vi "EC_Applied_Motion_SXSYSZ_20170419A_3chNoBKorg.vi"() -> ()   [LabVIEW 2015]
uses:
  <vilib>/Instr/_visa.llb/VISA Configure Serial Port (Instr).vi
  <userlib>/caLab/Private/Put_DBL-1D_PV-1D.vi
  <vilib>/Utility/file.llb/Write To Spreadsheet File (I64).vi
  <vilib>/Utility/file.llb/Read From Spreadsheet File (I64).vi
panel:
  in  "GFS":bool=TRUE
  out "NC":bool
  in  "Override 2":bool
  out "Dev5 Voltage 2":dbl
  out "Dev5 Voltage":dbl
  in  "Override":bool
  in  "APX:FZabs":dbl
  in  "Move Z":bool
  in  "Jog Z-":bool
  in  "Jog X-":bool
  in  "Jog Y-":bool
  out "Z Velocity MV mm/sec":dbl format="%.3f"
  out "Z Position MV mm":dbl
  out "Y Velocity MV mm/sec":dbl format="%.3f"
  out "Y Position MV mm":dbl
  out "X Velocity MV mm/sec":dbl format="%.3f"
  out "X Position MV mm":dbl
  in  "stop":bool
  in  "Tab Control 3":enum32{"Status", "Reset"}(tab)
  out "Y in Range":bool
  out "Y in Motion":bool
  out "X  in Range":bool
  out "X  in Motion":bool
  out "Z in Range":bool
  out "Z in Motion":bool
  out "X Ready":bool
  out "Y Ready":bool
  out "Z Ready":bool
  in  "Reset Y Position mm":dbl
  out "Reset Y Motor Steps":i32
  in  "Reset X Position mm":dbl
  out "Reset X Motor Steps":i32
  in  "Reset Z Position mm":dbl
  out "Reset Z Motor Steps":i32
  in  "Reset":bool
  in  "Tab Control":enum32{"mm", "preset", "step"}(tab)
  in  "APX:FXstep":dbl
  in  "FX Velocity SP mm/sec":dbl=0.01
  in  "APX:FYstep":dbl
  in  "FY Velocity SP mm/sec":dbl=0.01
  in  "APX:Fzstep":dbl
  in  "FZ Velocity SP mm/sec":dbl=0.01
  in  "Z Jog Set":bool
  in  "Y Jog Set":bool
  in  "X Jog Set":bool
  in  "X Velocity SP step/sec":i32 min=1 max=1000
  in  "Y Velocity SP step/sec":i32 min=1 max=1000
  in  "Z Velocity SP step/sec":i32 min=1 max=500
  in  "Y Step SP":i32=-20000 min=-800000 max=800000 step=500
  in  "X Step SP":i32=-20000 min=-750000 max=750000 step=500
  in  "Z Step SP":i32=-20000 min=-3000 max=102400000 step=500
  out "X Step PV":i32 max=2000
  out "Y Step PV":i32 max=2000
  out "Z Step PV":i32 max=2000
  out "R Step PV":i32 max=2000
  in  "Z Abso SP":i32=-20000 min=-3000 max=102400000 step=500
  out "Z COM PORT":refnum<visa-resource-name>="COM5"
  out "Z Holding Current %":i32
  out "Z Run Current %":i32
  out "Z offset mm":dbl
  out "Z mm/rev":dbl
  out "Z steps/rev":u32
  out "Z  velocity PV step/sec":i32
  out "Z MINPOS":i32=-94296
  out "Z MAXPOS":i32=-34296
  in  "Jog Z+":bool
  out "Z Position mm PV":dbl
  out "X Position mm PV":dbl
  out "X velocity PV step/sec":i32
  in  "Jog X+":bool
  out "X Holding Current %":i32
  out "X Run Current %":i32
  out "X offset mm":dbl
  out "X mm/rev":dbl
  out "X steps/rev":u32
  out "X MAXPOS":i32=-34296
  out "X MINPOS":i32=-94296
  out "X COM PORT":refnum<visa-resource-name>="COM5"
  out "Y Holding Current %":i32
  out "Y Run Current %":i32
  out "Y Position mm PV":dbl
  out "Y offset mm":dbl
  out "Y mm/rev":dbl
  out "Y steps/rev":u32
  out "Y velocity PV step/sec":i32
  in  "Stop":bool
  in  "Jog Y+":bool
  out "Y MINPOS":i32=-94296
  out "Y MAXPOS":i32=-34296
  out "Y COM PORT":refnum<visa-resource-name>="COM5"
  # "APX:FY"
  # "x-ray"
  # "APX:FZ"
  # "APX:FX"
  # "SPEAR"
  # "APX:FinePos"
  # "Stage"
  # "Current position"
  # "Jog step/velovity"
  # "sample to SSRL"
  # "FX"
  # "FY"
  # "FZ"
  # "R,L = green"
  # "L"
  # "M"
  # "B"
  # "S"
  # "R"
  # "Preset position"
types:
  T1 = enum16{"Power-up Signature", "Accel Rate", "Accel Max", "Bit Rate", "Buffer Status", "Change Current", "Commence Jogging", "Change Jog Speed", "Continue", "Define Address", "Distance for FC,FM,FO,FY", "Decel Rate", "Distance or Position", "Define Limits", "Encoder Deadband", "Encoder Function", "Encoder Position", "Encoder Ratio", "Feed to Length with Speed Change", "Feed to Length", "Feed to Sensor with Mask Dist", "Feed to Length & Set Output", "Feed to Position", "Feed to Sensor", "Feed to Sensor w/safety", "Follow Handwheel", "Immediate Distance?", "Immediate Encoder?", "Immediate Low Output", "Immediate High Output", "Immediate Position?", "Input Status?", "Jog Accel/Decel", "Jog Disable", "Jog Enable", "Jog Speed", "Motor Disable", "Motor Enable", "Microstep Resolution", "Power up Current", "Power up Mode", "Pause", "Request Status", "Revision Level?", "Seek Home", "Stop Jogging", "Stop & Kill Buffer", "Set Output", "Set ABS Position", "Send String", "Stop", "Velocity for Speed Change", "Velocity Setting", "Wait for Input", "Wait Time"}
  T2 = enum8{"Enabled", "Disabled", "Disabled and Grayed Out"}
  T3 = cluster{"first row[0]":i64, "first row[1]":i64, "first row[2]":i64, "first row[3]":i64, "first row[4]":i64, "first row[5]":i64, "first row[6]":i64, "first row[7]":i64, "first row[8]":i64}
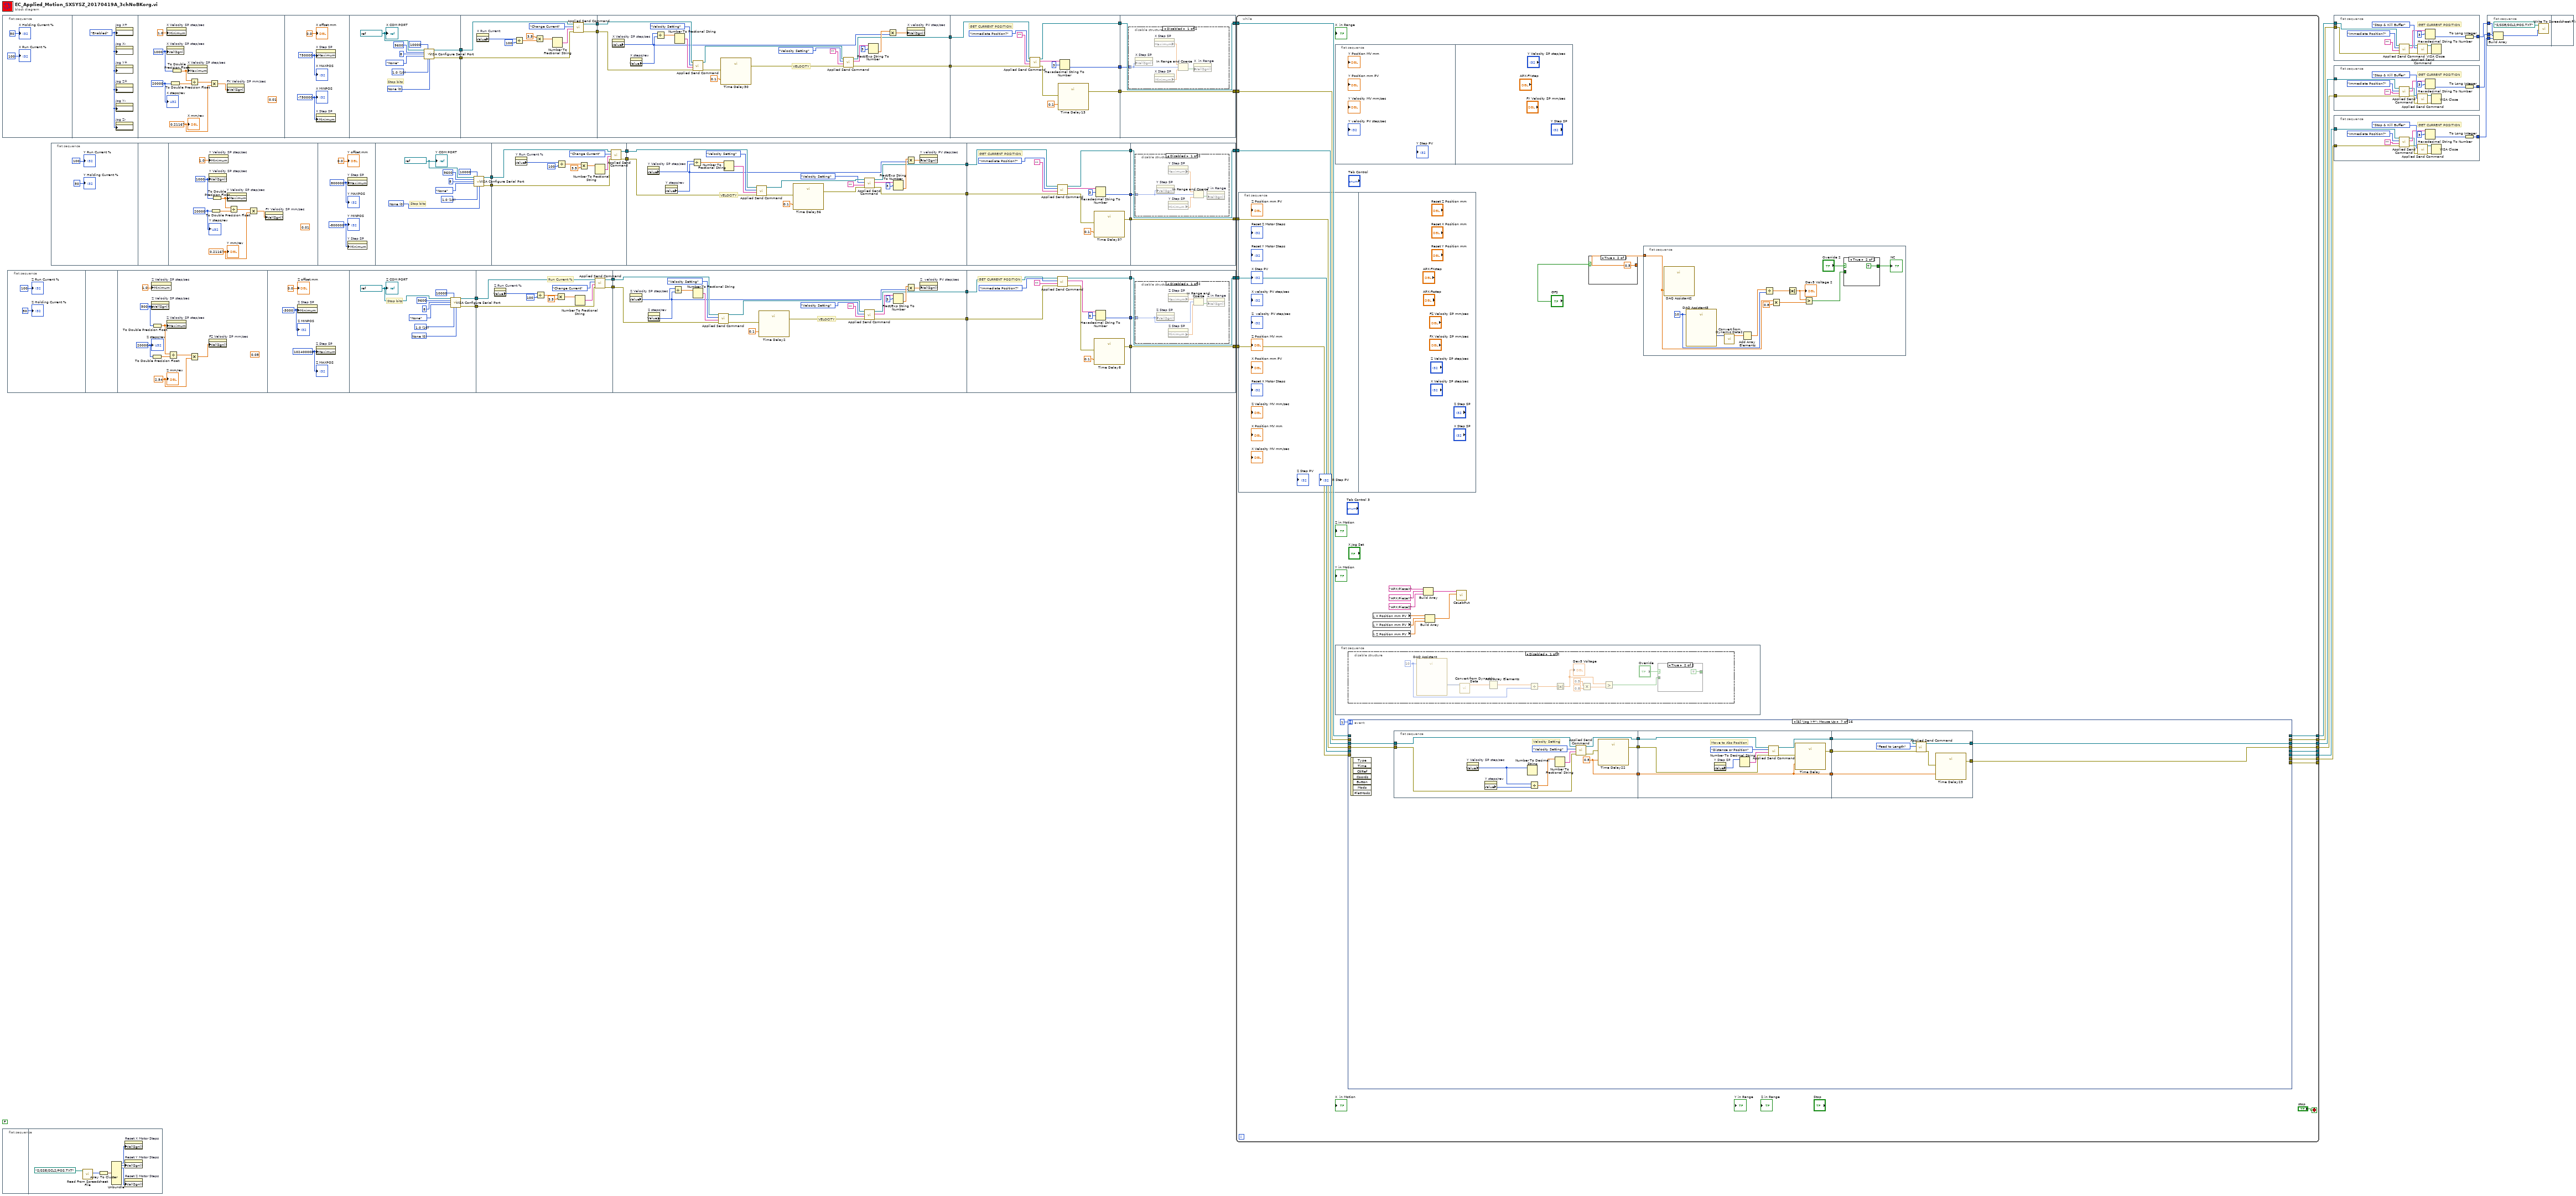
[diagram p0: block diagram]
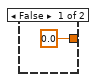
[diagram p5: hidden frame]
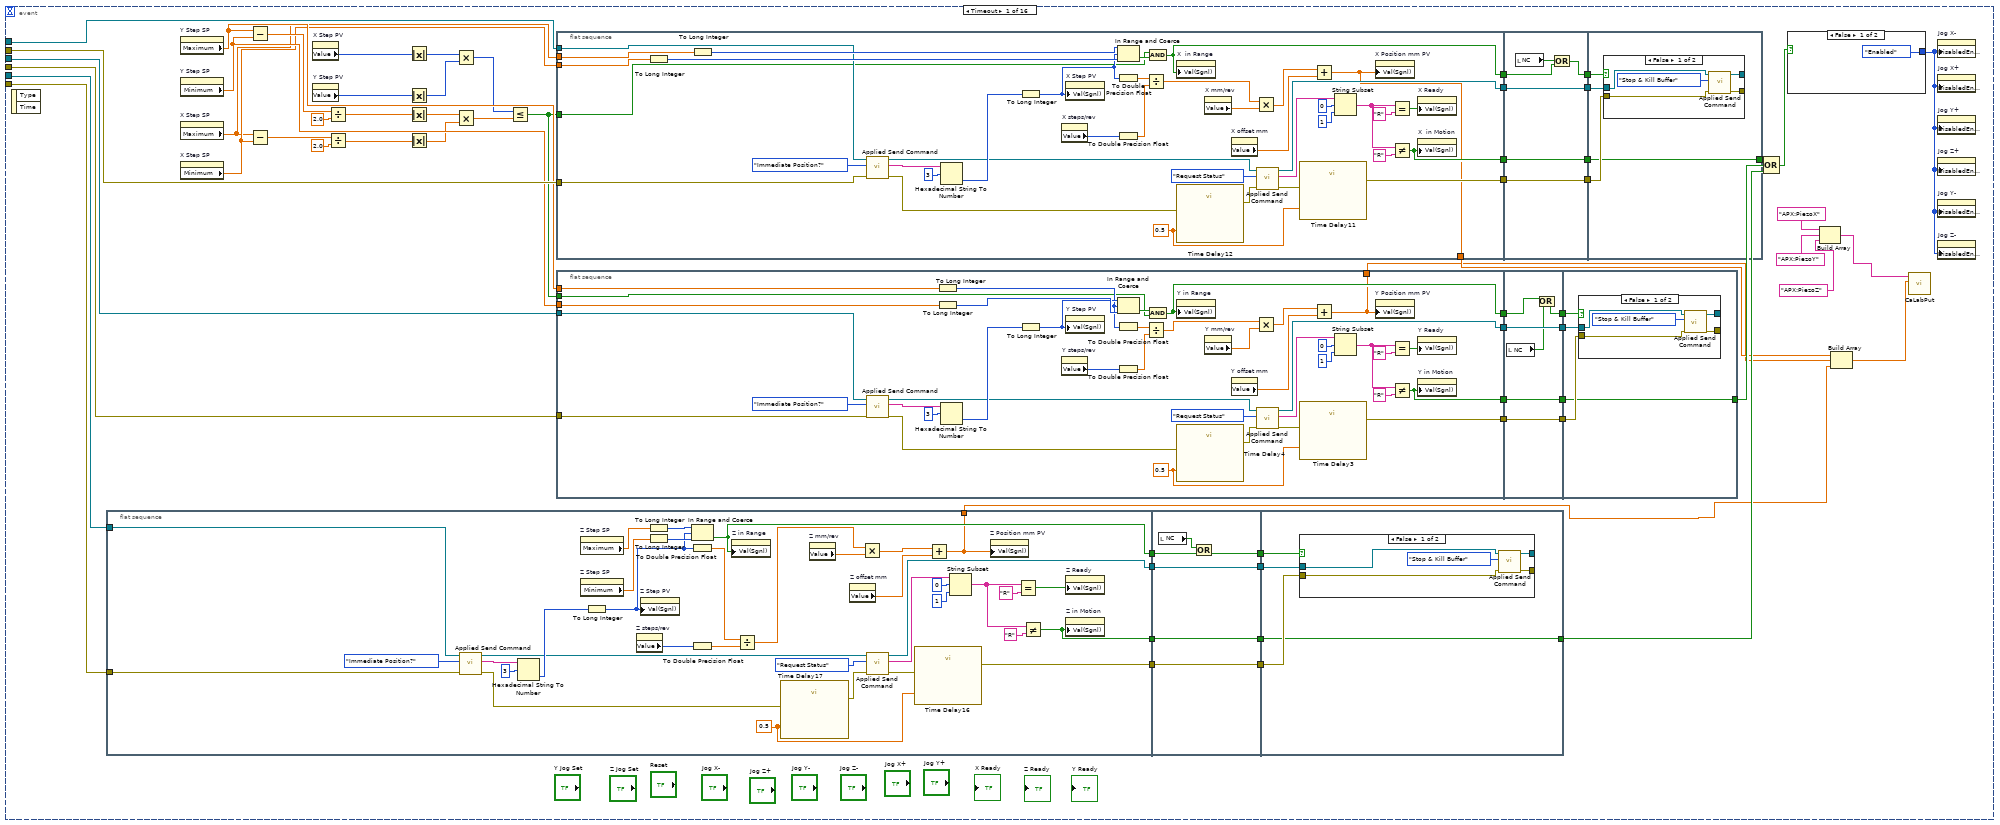
[diagram p9: hidden frame]
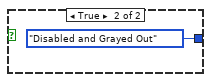
[diagram p10: hidden frame]
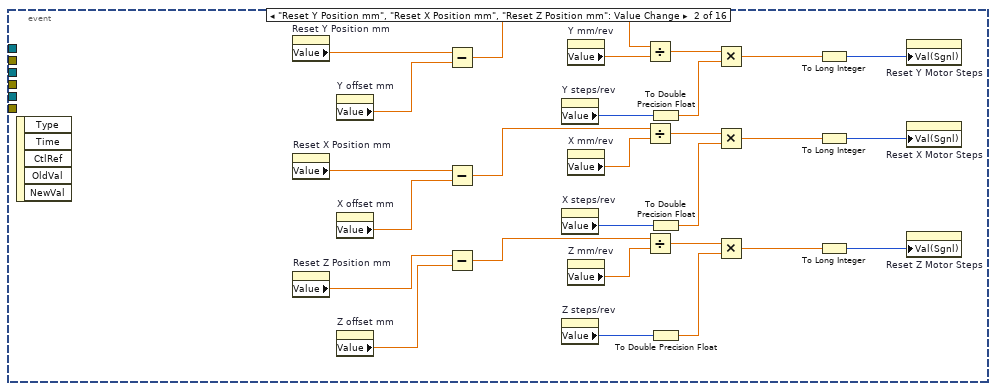
[diagram p14: hidden frame]
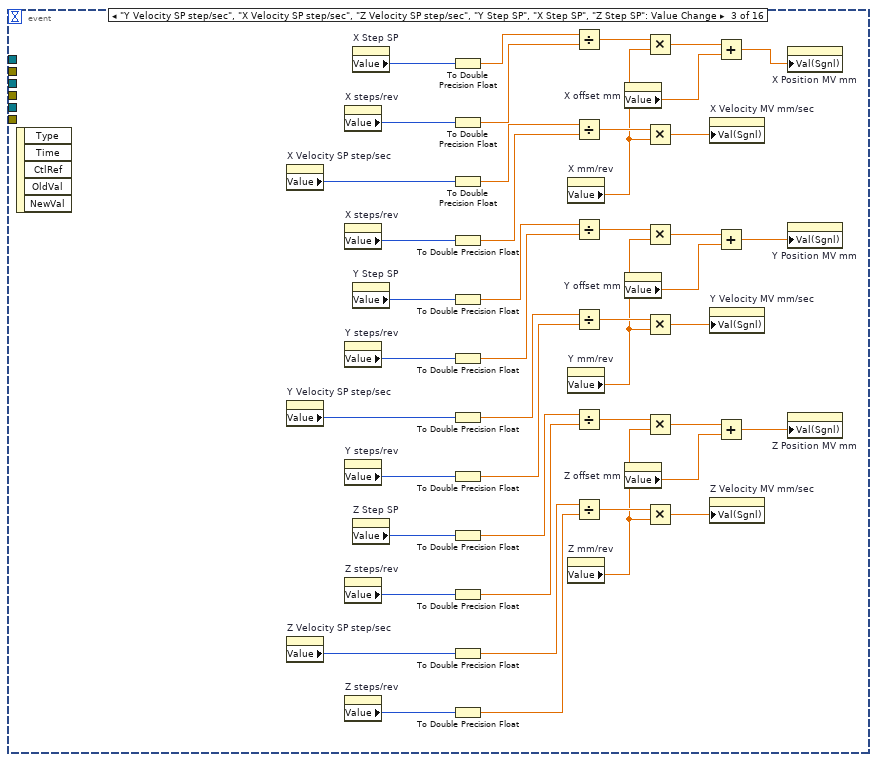
[diagram p15: hidden frame]
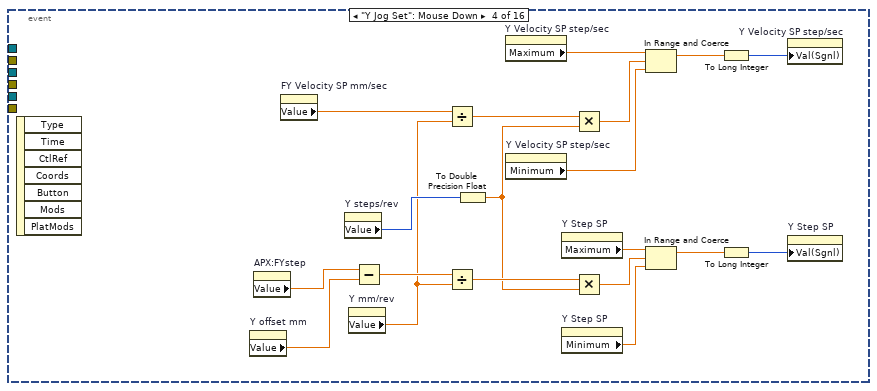
[diagram p16: hidden frame]
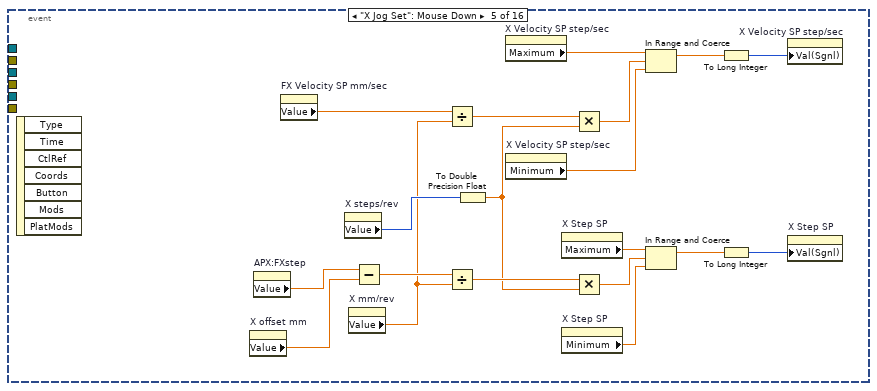
[diagram p17: hidden frame]
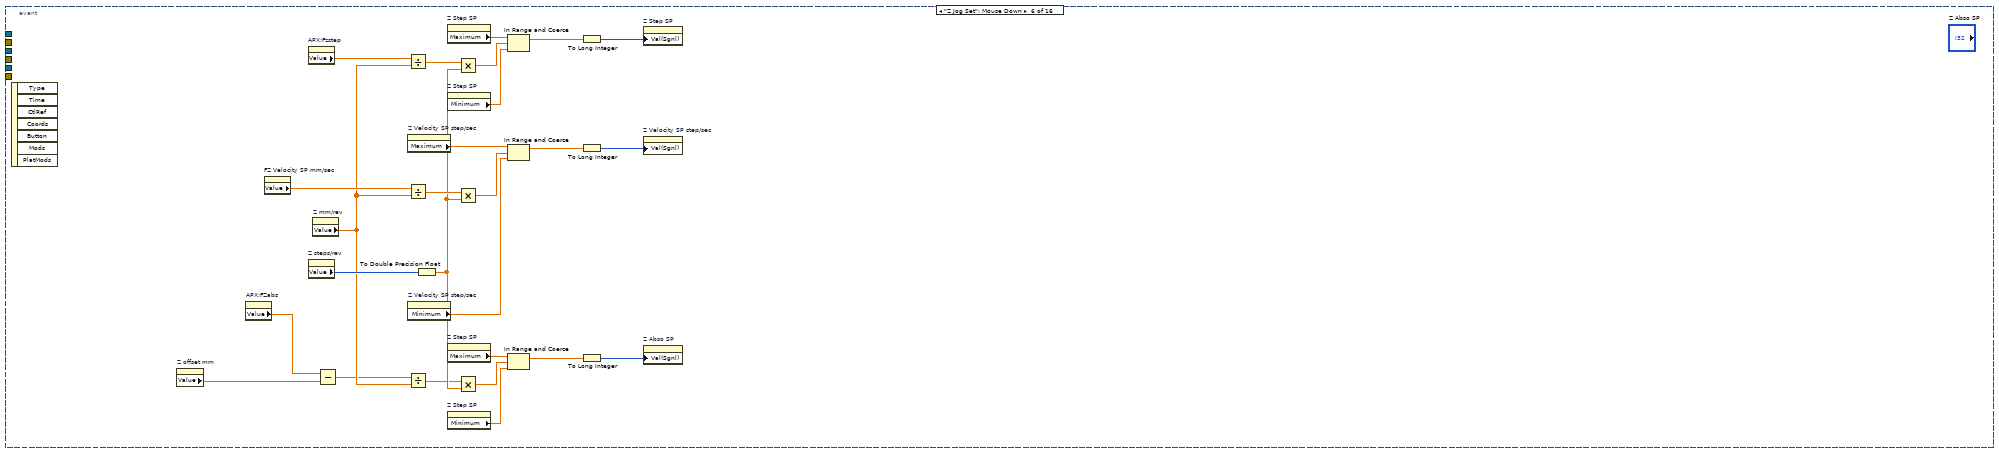
[diagram p18: hidden frame]
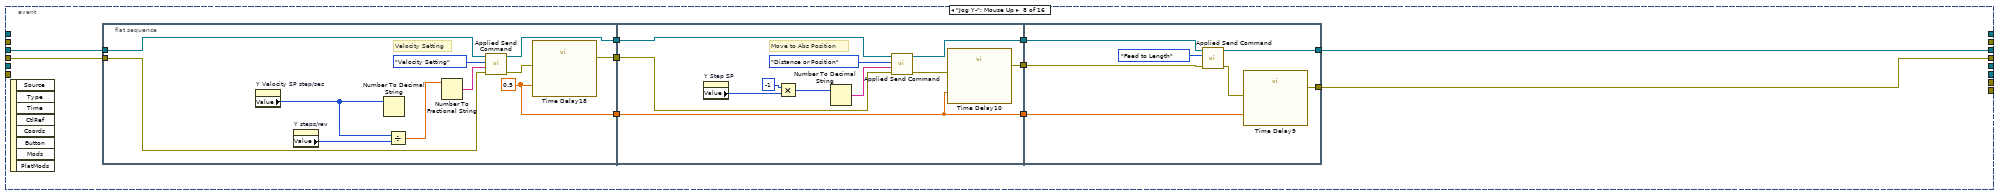
[diagram p19: hidden frame]
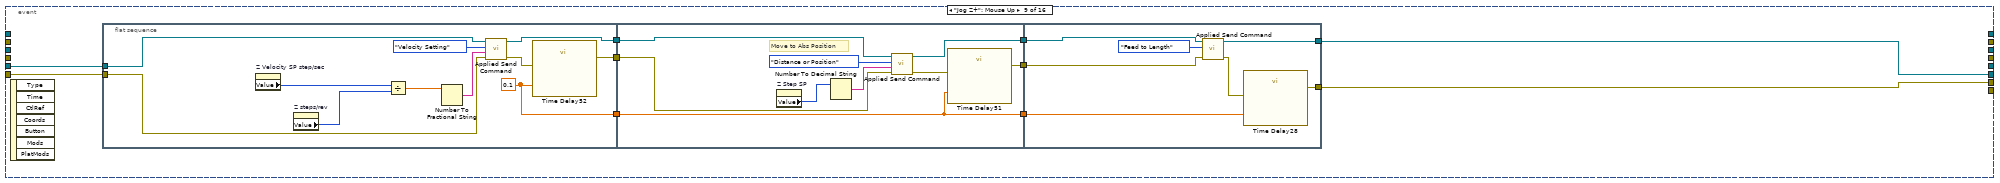
[diagram p20: hidden frame]
diagram:
  (unwired) FALSE
  n1 = flat-sequence {
    tunnel: [w58] -> w18
    tunnel: [w57] -> w17
    tunnel: w18 -> [w75]
    tunnel: w17 -> [w74]
    tunnel: [w73] -> w16
    tunnel: [w72] -> w15
    tunnel: [w78] -> w40
    tunnel: w16 -> [w86]
    tunnel: w15 -> [w85]
    tunnel: [w79] -> w14
    tunnel: w40 -> [w100]
    tunnel: [w99] -> w34
    tunnel: [w97] -> w33
    tunnel: [w102] -> w32
    tunnel: w14 -> [w101]
    tunnel: [w108] -> w38
    tunnel: [w109] -> w39
    tunnel: w34 -> [w109]
    tunnel: w33 -> [w108]
    tunnel: w32 -> [w107]
    frame #0 {
      "X Run Current %" <- 100 ("Run Current %")
      "X Holding Current %" <- 50 ("Holding Current %")
    }
    frame #1 {
      w45 = T2."Enabled" ("Disabled")
      n2 = property on="Jog X+" class="Bool"("DisabledEnum"=w45) -> ()  [unwired: 2 in, 2 out]
      n3 = property on="Jog X-" class="Bool"("DisabledEnum"=w45) -> ()  [unwired: 2 in, 2 out]
      n4 = property on="Jog Y+" class="Bool"("DisabledEnum"=w45) -> ()  [unwired: 2 in, 2 out]
      n5 = property on="Jog Z+" class="Bool"("DisabledEnum"=w45) -> ()  [unwired: 2 in, 2 out]
      n6 = property on="Jog Y-" class="Bool"("DisabledEnum"=w45) -> ()  [unwired: 2 in, 2 out]
      n7 = property on="Jog Z-" class="Bool"("DisabledEnum"=w45) -> ()  [unwired: 2 in, 2 out]
    }
    frame #2 {
      w48 = 0.21167 ("MM/rev")
      w51 = u32 20000 ("step/rev")
      w46 = 1000 ("Value (Signaling)")
      (unwired) 0.01 ("Value (Signaling)")
      n8 = property on="X Velocity SP step/sec" class="DigNum (strict)"("Minimum"=1.0 ("Data Entry Limits:Minimum")) -> ()  [unwired: 2 in, 2 out]
      n9 = property on="X Velocity SP step/sec" class="DigNum (strict)"("Val(Sgnl)"=w46) -> ()  [unwired: 2 in, 2 out]
      n10 = To Double Precision Float(number=w51) -> (double precision float=w50:dbl)
      n11 = To Double Precision Float(number=w46) -> (double precision float=w52:dbl)
      n12 = property on="X Velocity SP step/sec" class="DigNum (strict)"("Maximum"=w52) -> ()  [unwired: 2 in, 2 out]
      n13 = Divide(x=w52, y=w50) -> (x/y=w47:dbl)
      n14 = Multiply(x=w47, y=w48) -> (x*y=w49:dbl)
      n15 = property on="FX Velocity SP mm/sec" class="DigNum (strict)"("Val(Sgnl)"=w49) -> ()  [unwired: 2 in, 2 out]
      "X steps/rev" <- w51
      "X mm/rev" <- w48
    }
    frame #3 {
      w56 = -750000 ("lower limit")
      w55 = 750000 ("upper limit")
      n16 = property on="X Step SP" class="DigNum (strict)"("Maximum"=w55) -> ()  [unwired: 2 in, 2 out]
      n17 = property on="X Step SP" class="DigNum (strict)"("Minimum"=w56) -> ()  [unwired: 2 in, 2 out]
      "X offset mm" <- 0.0 ("offset")
      "X MAXPOS" <- w55
      "X MINPOS" <- w56
    }
    frame #4 {
      w65 = refnum<visa-resource-name> "COM21" ("COM PORT")
      w63 = u16 0 items=["None", "XON/XOFF", "RTS/CTS", "XON/XOFF & RTS/CTS", "DTR/DSR", "XON/XOFF & DTR/DSR"] ("flow control (0:none)")
      w62 = u16 10 items=["1.0"=10, "1.5"=15, "2.0"=20] ("stop bits (10: 1 bit)")
      # "Stop bits"
      n18 = call-poly "VISA Configure Serial Port"("VISA resource name"=w65, "timeout (10sec)"=u32 10000, "baud rate (9600)"=u32 9600, "data bits (8)"=u16 8, "parity (0:none)"=enum16{"None", "Odd", "Even", "Mark", "Space"}."None", "stop bits (10: 1 bit)"=w62, "flow control (0:none)"=w63) -> ("VISA resource name out"=w58:refnum<visa-resource-name>, "error out"=w57:errorcluster)  [unwired: 7 in]
      "X COM PORT" <- w65
    }
    frame #5 {
      n19 = property on="X Run Current" class="DigNum (strict)"() -> ("Value"=w70:i32)  [unwired: 2 in, 2 out]
      n20 = Divide(x=w70, y=100) -> (x/y=w67:dbl)
      n21 = Multiply(x=3.5 ("y"), y=w67) -> (x*y=w69:dbl)
      n22 = Number To Fractional String(number=w69) -> (F-format string=w71:string)  [unwired: 3 in]
      n23 = call "Applied Send Command.vi"("error in (no error)"=w74, "Extra"=w71, "Command"=T1."Change Current", "VISA resource name"=w75) -> ("error out"=w73:errorcluster, "VISA resource name out"=w72:refnum<visa-resource-name>)  [unwired: 3 in, 1 out]
    }
    frame #6 {
      # "VELOCITY"
      n24 = property on="X Velocity SP step/sec" class="DigNum (strict)"() -> ("Value"=w82:i32)  [unwired: 2 in, 2 out]
      n25 = property on="X steps/rev" class="DigNum (strict)"() -> ("Value"=w81:u32)  [unwired: 2 in, 2 out]
      n26 = Divide(x=w82, y=w81) -> (x/y=w80:dbl)
      n27 = Number To Fractional String(number=w80) -> (F-format string=w87:string)  [unwired: 3 in]
      n28 = call "Applied Send Command.vi"("error in (no error)"=w86, "Extra"=w87, "Command"=T1."Velocity Setting", "VISA resource name"=w85) -> ("error out"=w88:errorcluster, "VISA resource name out"=w95:refnum<visa-resource-name>)  [unwired: 3 in, 1 out]
      n29 = call "Time Delay30"("error in (no error)"=w88, "Delay Time (s)"=0.1) -> ("error out"=w93:errorcluster)  [unwired: 9 in]
      n30 = call "Applied Send Command.vi"("error in (no error)"=w93, "Extra"="", "Command"=T1."Velocity Setting", "VISA resource name"=w95) -> ("error out"=w78:errorcluster, "read buffer"=w91:string, "VISA resource name out"=w79:refnum<visa-resource-name>)  [unwired: 3 in]
      n31 = Fract/Exp String To Number(string=w91, offset=3) -> (number=w84:dbl)  [unwired: 2 in, 1 out]
      n32 = Multiply(x=w84, y=w81) -> (x*y=w83:dbl)
      n33 = property on="X velocity PV step/sec" class="DigNum (strict)"("Val(Sgnl)"=w83) -> ()  [unwired: 2 in, 2 out]
    }
    frame #7 {
      # "GET CURRENT POSITION"
      n34 = call "Applied Send Command.vi"("error in (no error)"=w100, "Extra"="", "Command"=T1."Immediate Position?", "VISA resource name"=w101) -> ("error out"=w98:errorcluster, "read buffer"=w104:string, "VISA resource name out"=w99:refnum<visa-resource-name>)  [unwired: 3 in]
      n35 = call "Time Delay13"("error in (no error)"=w98, "Delay Time (s)"=0.1) -> ("error out"=w97:errorcluster)  [unwired: 9 in]
      n36 = Hexadecimal String To Number(string=w104, offset=3) -> (number=w102:u32)  [unwired: 1 in, 1 out]
    }
    frame #8 {
      n37 = disable-structure shown="Disabled" {
        disable-tunnel: w107 -> [w110 _]
        frame Disabled {
          n38 = property on="X Step SP" class="DigNum (strict)"("Val(Sgnl)"=w110) -> ()  [unwired: 2 in, 2 out]
          n39 = property on="X Step SP" class="DigNum (strict)"() -> ("Maximum"=w113:dbl)  [unwired: 2 in, 2 out]
          n40 = property on="X Step SP" class="DigNum (strict)"() -> ("Minimum"=w112:dbl)  [unwired: 2 in, 2 out]
          n41 = In Range and Coerce(upper limit=w113, x=w110, lower limit=w112) -> (In Range?=w111:bool)  [unwired: 1 out]
          n42 = property on="X  in Range" class="Bool (strict)"("Val(Sgnl)"=w111) -> ()  [unwired: 2 in, 2 out]
        }
        frame Enabled {
        }
      }
    }
  }
  n43 = flat-sequence {
    frame #0 {
    }
    frame #1 {
      n44 = call-poly <vilib>:"Read From Spreadsheet File.vi"("file path (dialog if empty)"=path "S:/SSE/SCL2/POS.TXT") -> ("first row"=w114:i64[])  [unwired: 6 in, 4 out]
      n45 = Array To Cluster(array=w114) -> (cluster=w115:T3)
      n46 = Unbundle(w115) -> ("first row[0]"=w117:i64, "first row[1]"=w118:i64, "first row[2]"=w119:i64)  [unwired: 6 out]
      n47 = property on="Reset X Motor Steps" class="DigNum (strict)"("Val(Sgnl)"=w117) -> ()  [unwired: 2 in, 2 out]
      n48 = property on="Reset Y Motor Steps" class="DigNum (strict)"("Val(Sgnl)"=w118) -> ()  [unwired: 2 in, 2 out]
      n49 = property on="Reset Z Motor Steps" class="DigNum (strict)"("Val(Sgnl)"=w119) -> ()  [unwired: 2 in, 2 out]
    }
  }
  n50 = flat-sequence {
    tunnel: [w134] -> w5
    tunnel: [w133] -> w4
    tunnel: w5 -> [w148]
    tunnel: w4 -> [w147]
    tunnel: [w146] -> w3
    tunnel: [w145] -> w2
    tunnel: [w156] -> w31
    tunnel: [w155] -> w30
    tunnel: w3 -> [w158]
    tunnel: w2 -> [w157]
    tunnel: w31 -> [w173]
    tunnel: w30 -> [w172]
    tunnel: [w174] -> w29
    tunnel: [w175] -> w28
    tunnel: [w176] -> w1
    tunnel: [w184] -> w26
    tunnel: [w185] -> w27
    tunnel: w29 -> [w185]
    tunnel: w28 -> [w184]
    tunnel: w1 -> [w183]
    frame #0 {
      "Z Run Current %" <- 100 ("Z Run Current %")
      "Z Holding Current %" <- 50 ("Z Holding Current %")
    }
    frame #1 {
    }
    frame #2 {
      (unwired) 0.05 ("Value (Signaling)")
      w124 = 2.54 ("Z mm/rev")
      w123 = u32 20000 ("step/rev")
      w125 = 500 ("Value (Signaling)")
      n51 = property on="Z Velocity SP step/sec" class="DigNum (strict)"("Minimum"=1.0 ("Data Entry Limits:Minimum")) -> ()  [unwired: 2 in, 2 out]
      n52 = property on="Z Velocity SP step/sec" class="DigNum (strict)"("Val(Sgnl)"=w125) -> ()  [unwired: 2 in, 2 out]
      n53 = To Double Precision Float(number=w123) -> (double precision float=w128:dbl)
      n54 = To Double Precision Float(number=w125) -> (double precision float=w129:dbl)
      n55 = property on="Z Velocity SP step/sec" class="DigNum (strict)"("Maximum"=w129) -> ()  [unwired: 2 in, 2 out]
      n56 = Divide(x=w129, y=w128) -> (x/y=w126:dbl)
      n57 = Multiply(x=w126, y=w124) -> (x*y=w127:dbl)
      n58 = property on="FZ Velocity SP mm/sec" class="DigNum (strict)"("Val(Sgnl)"=w127) -> ()  [unwired: 2 in, 2 out]
      "Z mm/rev" <- w124
      "Z steps/rev" <- w123
    }
    frame #3 {
      w131 = -3000 ("lower limit")
      w130 = 102400000 ("upper limit")
      n59 = property on="Z Step SP" class="DigNum (strict)"("Minimum"=w131) -> ()  [unwired: 2 in, 2 out]
      n60 = property on="Z Step SP" class="DigNum (strict)"("Maximum"=w130) -> ()  [unwired: 2 in, 2 out]
      "Z offset mm" <- 0.0 ("Z offset mm")
      "Z MINPOS" <- w131
      "Z MAXPOS" <- w130
    }
    frame #4 {
      w141 = refnum<visa-resource-name> "COM23" ("COM PORT")
      w139 = u16 0 items=["None", "XON/XOFF", "RTS/CTS", "XON/XOFF & RTS/CTS", "DTR/DSR", "XON/XOFF & DTR/DSR"] ("flow control (0:none)")
      w138 = u16 10 items=["1.0"=10, "1.5"=15, "2.0"=20] ("stop bits (10: 1 bit)")
      # "Stop bits"
      n61 = call-poly "VISA Configure Serial Port"("VISA resource name"=w141, "timeout (10sec)"=u32 10000, "baud rate (9600)"=u32 9600, "data bits (8)"=u16 8, "parity (0:none)"=enum16{"None", "Odd", "Even", "Mark", "Space"}."None", "stop bits (10: 1 bit)"=w138, "flow control (0:none)"=w139) -> ("VISA resource name out"=w134:refnum<visa-resource-name>, "error out"=w133:errorcluster)  [unwired: 7 in]
      "Z COM PORT" <- w141
    }
    frame #5 {
      # "Run Current %"
      n62 = property on="Z Run Current %" class="DigNum (strict)"() -> ("Value"=w149:i32)  [unwired: 2 in, 2 out]
      n63 = Divide(x=w149, y=100) -> (x/y=w150:dbl)
      n64 = Multiply(x=w150, y=3.5) -> (x*y=w144:dbl)
      n65 = Number To Fractional String(number=w144) -> (F-format string=w151:string)  [unwired: 3 in]
      n66 = call "Applied Send Command.vi"("error in (no error)"=w147, "Extra"=w151, "Command"=T1."Change Current", "VISA resource name"=w148) -> ("error out"=w145:errorcluster, "VISA resource name out"=w146:refnum<visa-resource-name>)  [unwired: 3 in, 1 out]
    }
    frame #6 {
      # "VELOCITY"
      n67 = property on="Z Velocity SP step/sec" class="DigNum (strict)"() -> ("Value"=w153:i32)  [unwired: 2 in, 2 out]
      n68 = property on="Z steps/rev" class="DigNum (strict)"() -> ("Value"=w154:u32)  [unwired: 2 in, 2 out]
      n69 = Divide(x=w153, y=w154) -> (x/y=w161:dbl)
      n70 = Number To Fractional String(number=w161) -> (F-format string=w163:string)  [unwired: 3 in]
      n71 = call "Applied Send Command.vi"("error in (no error)"=w157, "Extra"=w163, "Command"=T1."Velocity Setting", "VISA resource name"=w158) -> ("error out"=w164:errorcluster, "VISA resource name out"=w171:refnum<visa-resource-name>)  [unwired: 3 in, 1 out]
      n72 = call "Time Delay2"("error in (no error)"=w164, "Delay Time (s)"=0.1) -> ("error out"=w169:errorcluster)  [unwired: 9 in]
      n73 = call "Applied Send Command.vi"("error in (no error)"=w169, "Extra"="", "Command"=T1."Velocity Setting", "VISA resource name"=w171) -> ("error out"=w155:errorcluster, "read buffer"=w167:string, "VISA resource name out"=w156:refnum<visa-resource-name>)  [unwired: 3 in]
      n74 = Fract/Exp String To Number(string=w167, offset=3) -> (number=w162:dbl)  [unwired: 2 in, 1 out]
      n75 = Multiply(x=w162, y=w154) -> (x*y=w159:dbl)
      n76 = property on="Z  velocity PV step/sec" class="DigNum (strict)"("Val(Sgnl)"=w159) -> ()  [unwired: 2 in, 2 out]
    }
    frame #7 {
      # "GET CURRENT POSITION"
      n77 = call "Applied Send Command.vi"("error in (no error)"=w172, "Extra"="", "Command"=T1."Immediate Position?", "VISA resource name"=w173) -> ("error out"=w178:errorcluster, "read buffer"=w180:string, "VISA resource name out"=w174:refnum<visa-resource-name>)  [unwired: 3 in]
      n78 = call "Time Delay8"("error in (no error)"=w178, "Delay Time (s)"=0.1) -> ("error out"=w175:errorcluster)  [unwired: 9 in]
      n79 = Hexadecimal String To Number(string=w180, offset=3) -> (number=w176:u32)  [unwired: 1 in, 1 out]
    }
    frame #8 {
      n80 = disable-structure shown="Disabled" {
        disable-tunnel: w183 -> [w188 _]
        frame Disabled {
          n81 = property on="Z Step SP" class="DigNum (strict)"("Val(Sgnl)"=w188) -> ()  [unwired: 2 in, 2 out]
          n82 = property on="Z Step SP" class="DigNum (strict)"() -> ("Maximum"=w187:dbl)  [unwired: 2 in, 2 out]
          n83 = property on="Z Step SP" class="DigNum (strict)"() -> ("Minimum"=w186:dbl)  [unwired: 2 in, 2 out]
          n84 = In Range and Coerce(upper limit=w187, x=w188, lower limit=w186) -> (In Range?=w189:bool)  [unwired: 1 out]
          n85 = property on="Z in Range" class="Bool (strict)"("Val(Sgnl)"=w189) -> ()  [unwired: 2 in, 2 out]
        }
        frame Enabled {
        }
      }
    }
  }
  n86 = flat-sequence {
    tunnel: [w204] -> w13
    tunnel: [w203] -> w12
    tunnel: w13 -> [w218]
    tunnel: w12 -> [w217]
    tunnel: [w216] -> w11
    tunnel: [w215] -> w10
    tunnel: w11 -> [w226]
    tunnel: w10 -> [w225]
    tunnel: [w224] -> w9
    tunnel: [w223] -> w8
    tunnel: [w243] -> w35
    tunnel: w9 -> [w246]
    tunnel: w8 -> [w245]
    tunnel: [w244] -> w7
    tunnel: [w242] -> w6
    tunnel: [w253] -> w41
    tunnel: [w255] -> w42
    tunnel: w35 -> [w253]
    tunnel: w7 -> [w255]
    tunnel: w6 -> [w254]
    frame #0 {
      "Y Run Current %" <- 100 ("Run Current %")
      "Y Holding Current %" <- 50 ("Holding Current %")
    }
    frame #1 {
    }
    frame #2 {
      w194 = 0.21167 ("MM/rev")
      w197 = u32 20000 ("step/rev")
      w192 = 1000 ("Value (Signaling)")
      (unwired) 0.01 ("Value (Signaling)")
      n87 = property on="Y Velocity SP step/sec" class="DigNum (strict)"("Minimum"=1.0 ("Data Entry Limits:Minimum")) -> ()  [unwired: 2 in, 2 out]
      n88 = property on="Y Velocity SP step/sec" class="DigNum (strict)"("Val(Sgnl)"=w192) -> ()  [unwired: 2 in, 2 out]
      n89 = To Double Precision Float(number=w197) -> (double precision float=w196:dbl)
      n90 = To Double Precision Float(number=w192) -> (double precision float=w198:dbl)
      n91 = property on="Y Velocity SP step/sec" class="DigNum (strict)"("Maximum"=w198) -> ()  [unwired: 2 in, 2 out]
      n92 = Divide(x=w198, y=w196) -> (x/y=w193:dbl)
      n93 = Multiply(x=w193, y=w194) -> (x*y=w195:dbl)
      n94 = property on="FY Velocity SP mm/sec" class="DigNum (strict)"("Val(Sgnl)"=w195) -> ()  [unwired: 2 in, 2 out]
      "Y steps/rev" <- w197
      "Y mm/rev" <- w194
    }
    frame #3 {
      w201 = -800000 ("lower limit")
      w202 = 800000 ("upper limit")
      n95 = property on="Y Step SP" class="DigNum (strict)"("Maximum"=w202) -> ()  [unwired: 2 in, 2 out]
      n96 = property on="Y Step SP" class="DigNum (strict)"("Minimum"=w201) -> ()  [unwired: 2 in, 2 out]
      "Y MAXPOS" <- w202
      "Y MINPOS" <- w201
      "Y offset mm" <- 0.0 ("offset")
    }
    frame #4 {
      w211 = refnum<visa-resource-name> "COM22" ("COM PORT")
      w209 = u16 0 items=["None", "XON/XOFF", "RTS/CTS", "XON/XOFF & RTS/CTS", "DTR/DSR", "XON/XOFF & DTR/DSR"] ("flow control (0:none)")
      w208 = u16 10 items=["1.0"=10, "1.5"=15, "2.0"=20] ("stop bits (10: 1 bit)")
      # "Stop bits"
      n97 = call-poly "VISA Configure Serial Port"("VISA resource name"=w211, "timeout (10sec)"=u32 10000, "baud rate (9600)"=u32 9600, "data bits (8)"=u16 8, "parity (0:none)"=enum16{"None", "Odd", "Even", "Mark", "Space"}."None", "stop bits (10: 1 bit)"=w208, "flow control (0:none)"=w209) -> ("VISA resource name out"=w204:refnum<visa-resource-name>, "error out"=w203:errorcluster)  [unwired: 7 in]
      "Y COM PORT" <- w211
    }
    frame #5 {
      n98 = property on="Y Run Current %" class="DigNum (strict)"() -> ("Value"=w219:i32)  [unwired: 2 in, 2 out]
      n99 = Divide(x=w219, y=100) -> (x/y=w220:dbl)
      n100 = Multiply(x=w220, y=3.5) -> (x*y=w214:dbl)
      n101 = Number To Fractional String(number=w214) -> (F-format string=w221:string)  [unwired: 3 in]
      n102 = call "Applied Send Command.vi"("error in (no error)"=w217, "Extra"=w221, "Command"=T1."Change Current", "VISA resource name"=w218) -> ("error out"=w215:errorcluster, "VISA resource name out"=w216:refnum<visa-resource-name>)  [unwired: 3 in, 1 out]
    }
    frame #6 {
      # "VELOCITY"
      n103 = property on="Y Velocity SP step/sec" class="DigNum (strict)"() -> ("Value"=w227:i32)  [unwired: 2 in, 2 out]
      n104 = property on="Y steps/rev" class="DigNum (strict)"() -> ("Value"=w230:u32)  [unwired: 2 in, 2 out]
      n105 = Divide(x=w227, y=w230) -> (x/y=w229:dbl)
      n106 = Number To Fractional String(number=w229) -> (F-format string=w233:string)  [unwired: 3 in]
      n107 = call "Applied Send Command.vi"("error in (no error)"=w225, "Extra"=w233, "Command"=T1."Velocity Setting", "VISA resource name"=w226) -> ("error out"=w234:errorcluster, "VISA resource name out"=w241:refnum<visa-resource-name>)  [unwired: 3 in, 1 out]
      n108 = call "Time Delay36"("error in (no error)"=w234, "Delay Time (s)"=0.1) -> ("error out"=w239:errorcluster)  [unwired: 9 in]
      n109 = call "Applied Send Command.vi"("error in (no error)"=w239, "Extra"="", "Command"=T1."Velocity Setting", "VISA resource name"=w241) -> ("error out"=w223:errorcluster, "read buffer"=w237:string, "VISA resource name out"=w224:refnum<visa-resource-name>)  [unwired: 3 in]
      n110 = Fract/Exp String To Number(string=w237, offset=3) -> (number=w232:dbl)  [unwired: 2 in, 1 out]
      n111 = Multiply(x=w232, y=w230) -> (x*y=w231:dbl)
      n112 = property on="Y velocity PV step/sec" class="DigNum (strict)"("Val(Sgnl)"=w231) -> ()  [unwired: 2 in, 2 out]
    }
    frame #7 {
      # "GET CURRENT POSITION"
      n113 = call "Applied Send Command.vi"("error in (no error)"=w245, "Extra"="", "Command"=T1."Immediate Position?", "VISA resource name"=w246) -> ("error out"=w248:errorcluster, "read buffer"=w250:string, "VISA resource name out"=w244:refnum<visa-resource-name>)  [unwired: 3 in]
      n114 = call "Time Delay37"("error in (no error)"=w248, "Delay Time (s)"=0.1) -> ("error out"=w243:errorcluster)  [unwired: 9 in]
      n115 = Hexadecimal String To Number(string=w250, offset=3) -> (number=w242:u32)  [unwired: 1 in, 1 out]
    }
    frame #8 {
      n116 = disable-structure shown="Disabled" {
        disable-tunnel: w254 -> [w258 _]
        frame Disabled {
          n117 = property on="Y Step SP" class="DigNum (strict)"("Val(Sgnl)"=w258) -> ()  [unwired: 2 in, 2 out]
          n118 = property on="Y Step SP" class="DigNum (strict)"() -> ("Maximum"=w257:dbl)  [unwired: 2 in, 2 out]
          n119 = property on="Y Step SP" class="DigNum (strict)"() -> ("Minimum"=w256:dbl)  [unwired: 2 in, 2 out]
          n120 = In Range and Coerce(upper limit=w257, x=w258, lower limit=w256) -> (In Range?=w259:bool)  [unwired: 1 out]
          n121 = property on="Y in Range" class="Bool (strict)"("Val(Sgnl)"=w259) -> ()  [unwired: 2 in, 2 out]
        }
        frame Enabled {
        }
      }
    }
  }
  n122 = while {
    tunnel: w42 -> [w281]
    tunnel: w41 -> [w284]
    tunnel: [w285] -> w22
    tunnel: [w283] -> w23
    tunnel: w39 -> [w280]
    tunnel: w38 -> [w279]
    tunnel: [w278] -> w37
    tunnel: [w277] -> w36
    tunnel: w27 -> [w276]
    tunnel: w26 -> [w275]
    tunnel: [w274] -> w25
    tunnel: [w273] -> w24
    tunnel: [w272] -> _
    tunnel: [w271] -> _
    stop <- "stop" stop-if-true
    n123 = flat-sequence {
      frame #0 {
      }
      frame #1 {
      }
    }
    n124 = flat-sequence {
      frame #0 {
      }
      frame #1 {
      }
    }
    n125 = flat-sequence {
      frame #0 {
        n126 = disable-structure shown="Disabled" {
          frame Disabled {
            w303 = 10 ("number of samples")
            n127 = call "DAQ Assistant"("number of samples"=w303) -> ("data"=w308:dynamicdata)  [unwired: 16 in, 2 out]
            n128 = call "Convert from Dynamic Data"("Dynamic Data Type"=w308) -> ("Array"=w309:dbl[])  [unwired: 3 in]
            n129 = Add Array Elements(numeric array=w309) -> (sum=w307:dbl)
            n130 = Divide(x=w307, y=w303) -> (x/y=w306:dbl)
            n131 = Absolute Value(x=w306) -> (abs(x)=w310:dbl)
            "Dev5 Voltage" <- w310
            n132 = Multiply(x=0.5, y=0.8) -> (x*y=w304:dbl)
            n133 = Greater?(x=w310, y=w304) -> (0:w311:bool)
            n134 = case shown="True" "Override" {
              tunnel: [w313 TRUE] -> _
              tunnel: w311 -> [w313 _]
              frame False {
              }
              frame True {
              }
            }
          }
          frame Enabled {
          }
        }
      }
    }
    n135 = event shown="[6] \"Jog Y+\": Mouse Up" {
      selector: _ -> [_ _ _ _ _ _ _ _ _ _ _ _ _ _ _ _]
      dyn-events: _ -> [_ _ _ _ _ _ _ _ _ _ _ _ _ _ _ _]
      timeout: 1 -> [_ _ _ _ _ _ _ _ _ _ _ _ _ _ _ _]
      tunnel: w284 -> [w376 _ _ _ _ _ w680 w717 _ _ _ _ _ w943 w955 w982]
      tunnel: [_ _ _ _ _ _ w686 w723 _ _ _ _ _ w943 w953 w980] -> w285
      tunnel: w281 -> [w348 _ _ _ _ _ w681 w718 _ _ _ _ _ w944 w956 w983]
      tunnel: [_ _ _ _ _ _ w687 w724 _ _ _ _ _ w944 w954 w981] -> w283
      tunnel: w280 -> [w347 _ _ _ _ _ _ _ _ _ _ w876 w913 _ w950 w979]
      tunnel: w279 -> [w359 _ _ _ _ _ _ _ _ _ _ w875 w912 _ w949 w978]
      tunnel: [_ _ _ _ _ _ _ _ _ _ _ w874 w911 _ w952 w977] -> w278
      tunnel: [_ _ _ _ _ _ _ _ _ _ _ w873 w910 _ w951 w976] -> w277
      tunnel: w276 -> [w349 _ _ _ _ _ _ _ w759 w796 w833 _ _ _ w948 w975]
      tunnel: w275 -> [w350 _ _ _ _ _ _ _ w758 w795 w832 _ _ _ w947 w974]
      tunnel: [_ _ _ _ _ _ _ _ w756 w793 w830 _ _ _ w946 _] -> w274
      tunnel: [_ _ _ _ _ _ _ _ w757 w794 w831 _ _ _ w945 _] -> w273
      tunnel: [_ _ _ _ _ _ _ _ _ _ _ _ _ _ _ w973] -> w272
      tunnel: [_ _ _ _ _ _ _ _ _ _ _ _ _ _ _ w972] -> w271
      event Timeout {
        n136 = event-data() -> ()  [unwired: 1 in, 2 out]
        n137 = flat-sequence {
          tunnel: [w388] -> w358
          tunnel: [w401] -> w357
          tunnel: [w410] -> w356
          tunnel: [w381] -> w355
          tunnel: w349 -> [w396]
          tunnel: w350 -> [w397]
          tunnel: [w379] -> w316
          tunnel: w358 -> [w420]
          tunnel: [w420] -> w354
          tunnel: w357 -> [w419]
          tunnel: [w419] -> w353
          tunnel: w356 -> [w418]
          tunnel: [w416] -> w352
          tunnel: w355 -> [w417]
          tunnel: [w417] -> w351
          tunnel: w354 -> [w423]
          tunnel: w353 -> [w424]
          tunnel: w352 -> [w422]
          tunnel: w351 -> [w421]
          tunnel: [w421] -> w324
          frame #0 {
            w400 = 0.5 ("Delay Time (s)")
            n138 = call "Applied Send Command.vi"("error in (no error)"=w397, "Command"=T1."Immediate Position?", "VISA resource name"=w396) -> ("error out"=w395:errorcluster, "read buffer"=w392:string, "VISA resource name out"=w390:refnum<visa-resource-name>)  [unwired: 4 in]
            n139 = Hexadecimal String To Number(string=w392, offset=3) -> (number=w393:u32)  [unwired: 1 in, 1 out]
            n140 = property on="Z Step SP" class="DigNum (strict)"() -> ("Maximum"=w412:dbl)  [unwired: 2 in, 2 out]
            n141 = property on="Z Step SP" class="DigNum (strict)"() -> ("Minimum"=w414:dbl)  [unwired: 2 in, 2 out]
            n142 = To Long Integer(number=w393) -> (32bit integer=w402:i32)
            n143 = property on="Z steps/rev" class="DigNum (strict)"() -> ("Value"=w408:u32)  [unwired: 2 in, 2 out]
            n144 = property on="Z Step PV" class="DigNum (strict)"("Val(Sgnl)"=w402) -> ()  [unwired: 2 in, 2 out]
            n145 = To Long Integer(number=w412) -> (32bit integer=w411:i32)
            n146 = To Long Integer(number=w414) -> (32bit integer=w413:i32)
            n147 = In Range and Coerce(upper limit=w411, x=w402, lower limit=w413) -> (In Range?=w410:bool)  [unwired: 1 out]
            n148 = To Double Precision Float(number=w402) -> (double precision float=w403:dbl)
            n149 = To Double Precision Float(number=w408) -> (double precision float=w409:dbl)
            n150 = property on="Z in Range" class="Bool (strict)"("Val(Sgnl)"=w410) -> ()  [unwired: 2 in, 2 out]
            n151 = Divide(x=w403, y=w409) -> (x/y=w407:dbl)
            n152 = call "Time Delay17"("error in (no error)"=w395, "Delay Time (s)"=w400) -> ("error out"=w380:errorcluster)  [unwired: 9 in]
            n153 = property on="Z mm/rev" class="DigNum (strict)"() -> ("Value"=w406:dbl)  [unwired: 2 in, 2 out]
            n154 = property on="Z offset mm" class="DigNum (strict)"() -> ("Value"=w404:dbl)  [unwired: 2 in, 2 out]
            n155 = Multiply(x=w407, y=w406) -> (x*y=w405:dbl)
            n156 = call "Applied Send Command.vi"("error in (no error)"=w380, "Command"=T1."Request Status", "VISA resource name"=w390) -> ("error out"=w389:errorcluster, "read buffer"=w385:string, "VISA resource name out"=w388:refnum<visa-resource-name>)  [unwired: 4 in]
            n157 = call "Time Delay16"("error in (no error)"=w389, "Delay Time (s)"=w400) -> ("error out"=w401:errorcluster)  [unwired: 9 in]
            n158 = Add(x=w405, y=w404) -> (x+y=w379:dbl)
            n159 = String Subset(string=w385, offset (0)=0, length (rest)=1 ("length (rest)")) -> (substring=w382:string)
            n160 = property on="Z Position mm PV" class="DigNum (strict)"("Val(Sgnl)"=w379) -> ()  [unwired: 2 in, 2 out]
            n161 = Equal?(x=w382, y="R") -> (x = y?=w399:bool)
            n162 = Not Equal?(x=w382, y="R") -> (x != y?=w381:bool)
            n163 = property on="Z Ready" class="Bool (strict)"("Val(Sgnl)"=w399) -> ()  [unwired: 2 in, 2 out]
            n164 = property on="Z in Motion" class="Bool (strict)"("Val(Sgnl)"=w381) -> ()  [unwired: 2 in, 2 out]
          }
          frame #1 {
            n165 = local read "NC"() -> (w415:bool)
            n166 = Or(x=w415, y=w418) -> (x .or. y?=w416:bool)
          }
          frame #2 {
            n167 = case shown="False" w422 {
              tunnel: w423 -> [w428 w431]
              tunnel: [w426 w431] -> _
              tunnel: [w425 w430] -> _
              tunnel: w424 -> [w427 w430]
              frame False {
                n168 = call "Applied Send Command.vi"("error in (no error)"=w427, "Command"=T1."Stop & Kill Buffer", "VISA resource name"=w428) -> ("error out"=w425:errorcluster, "VISA resource name out"=w426:refnum<visa-resource-name>)  [unwired: 4 in, 1 out]
              }
              frame True {
              }
            }
          }
        }
        n169 = property on="Y Step SP" class="DigNum (strict)"() -> ("Maximum"=w344:dbl)  [unwired: 2 in, 2 out]
        n170 = property on="Y Step SP" class="DigNum (strict)"() -> ("Minimum"=w343:dbl)  [unwired: 2 in, 2 out]
        n171 = property on="X Step SP" class="DigNum (strict)"() -> ("Maximum"=w339:dbl)  [unwired: 2 in, 2 out]
        n172 = property on="X Step SP" class="DigNum (strict)"() -> ("Minimum"=w340:dbl)  [unwired: 2 in, 2 out]
        n173 = Subtract(x=w344, y=w343) -> (x-y=w345:dbl)
        n174 = Subtract(x=w339, y=w340) -> (x-y=w341:dbl)
        n175 = property on="X Step PV" class="DigNum (strict)"() -> ("Value"=w338:i32)  [unwired: 2 in, 2 out]
        n176 = property on="Y Step PV" class="DigNum (strict)"() -> ("Value"=w337:i32)  [unwired: 2 in, 2 out]
        n177 = Divide(x=w345, y=2.0) -> (x/y=w333:dbl)
        n178 = Divide(x=w341, y=2.0) -> (x/y=w334:dbl)
        n179 = Absolute Value(x=w338) -> (abs(x)=w335:i32)
        n180 = Absolute Value(x=w337) -> (abs(x)=w336:i32)
        n181 = Absolute Value(x=w333) -> (abs(x)=w331:dbl)
        n182 = Absolute Value(x=w334) -> (abs(x)=w332:dbl)
        n183 = Multiply(x=w335, y=w336) -> (x*y=w330:i32)
        n184 = Multiply(x=w331, y=w332) -> (x*y=w329:dbl)
        n185 = Less Or Equal?(x=w330, y=w329) -> (x <= y?=w328:bool)
        n186 = flat-sequence {
          tunnel: [w445] -> w367
          tunnel: [w456] -> w366
          tunnel: [w434] -> w365
          tunnel: [w441] -> w364
          tunnel: w347 -> [w452]
          tunnel: w359 -> [w440]
          tunnel: w339 -> [w436]
          tunnel: w340 -> [w435]
          tunnel: w328 -> [w433]
          tunnel: [w432] -> w318
          tunnel: w367 -> [w475]
          tunnel: [w475] -> w363
          tunnel: w366 -> [w474]
          tunnel: [w474] -> w362
          tunnel: w365 -> [w471]
          tunnel: [w470] -> w361
          tunnel: w364 -> [w473]
          tunnel: [w473] -> w360
          tunnel: w363 -> [w479]
          tunnel: w362 -> [w478]
          tunnel: w361 -> [w477]
          tunnel: w360 -> [w476]
          tunnel: [w476] -> w326
          frame #0 {
            w455 = 0.5 ("Delay Time (s)")
            n187 = To Long Integer(number=w435) -> (32bit integer=w468:i32)
            n188 = To Long Integer(number=w436) -> (32bit integer=w467:i32)
            n189 = call "Applied Send Command.vi"("error in (no error)"=w440, "Command"=T1."Immediate Position?", "VISA resource name"=w452) -> ("error out"=w450:errorcluster, "read buffer"=w451:string, "VISA resource name out"=w446:refnum<visa-resource-name>)  [unwired: 4 in]
            n190 = Hexadecimal String To Number(string=w451, offset=3) -> (number=w457:u32)  [unwired: 1 in, 1 out]
            n191 = To Long Integer(number=w457) -> (32bit integer=w458:i32)
            n192 = property on="X steps/rev" class="DigNum (strict)"() -> ("Value"=w464:u32)  [unwired: 2 in, 2 out]
            n193 = property on="X Step PV" class="DigNum (strict)"("Val(Sgnl)"=w458) -> ()  [unwired: 2 in, 2 out]
            n194 = In Range and Coerce(upper limit=w467, x=w458, lower limit=w468) -> (In Range?=w466:bool)  [unwired: 1 out]
            n195 = To Double Precision Float(number=w458) -> (double precision float=w459:dbl)
            n196 = To Double Precision Float(number=w464) -> (double precision float=w465:dbl)
            n197 = Divide(x=w459, y=w465) -> (x/y=w463:dbl)
            n198 = And(x=w433, y=w466) -> (x .and. y?=w434:bool)
            n199 = property on="X  in Range" class="Bool (strict)"("Val(Sgnl)"=w434) -> ()  [unwired: 2 in, 2 out]
            n200 = call "Time Delay12"("error in (no error)"=w450, "Delay Time (s)"=w455) -> ("error out"=w443:errorcluster)  [unwired: 9 in]
            n201 = property on="X mm/rev" class="DigNum (strict)"() -> ("Value"=w462:dbl)  [unwired: 2 in, 2 out]
            n202 = property on="X offset mm" class="DigNum (strict)"() -> ("Value"=w460:dbl)  [unwired: 2 in, 2 out]
            n203 = Multiply(x=w463, y=w462) -> (x*y=w461:dbl)
            n204 = call "Applied Send Command.vi"("error in (no error)"=w443, "Command"=T1."Request Status", "VISA resource name"=w446) -> ("error out"=w444:errorcluster, "read buffer"=w448:string, "VISA resource name out"=w445:refnum<visa-resource-name>)  [unwired: 4 in]
            n205 = call "Time Delay11"("error in (no error)"=w444, "Delay Time (s)"=w455) -> ("error out"=w456:errorcluster)  [unwired: 9 in]
            n206 = Add(x=w461, y=w460) -> (x+y=w432:dbl)
            n207 = String Subset(string=w448, offset (0)=0, length (rest)=1 ("length (rest)")) -> (substring=w437:string)
            n208 = property on="X Position mm PV" class="DigNum (strict)"("Val(Sgnl)"=w432) -> ()  [unwired: 2 in, 2 out]
            n209 = Equal?(x=w437, y="R") -> (x = y?=w454:bool)
            n210 = Not Equal?(x=w437, y="R") -> (x != y?=w441:bool)
            n211 = property on="X Ready" class="Bool (strict)"("Val(Sgnl)"=w454) -> ()  [unwired: 2 in, 2 out]
            n212 = property on="X  in Motion" class="Bool (strict)"("Val(Sgnl)"=w441) -> ()  [unwired: 2 in, 2 out]
          }
          frame #1 {
            n213 = local read "NC"() -> (w472:bool)
            n214 = Or(x=w472, y=w471) -> (x .or. y?=w470:bool)
          }
          frame #2 {
            n215 = case shown="False" w477 {
              tunnel: w479 -> [w481 w486]
              tunnel: [w483 w486] -> _
              tunnel: [w484 w485] -> _
              tunnel: w478 -> [w480 w485]
              frame False {
                n216 = call "Applied Send Command.vi"("error in (no error)"=w480, "Command"=T1."Stop & Kill Buffer", "VISA resource name"=w481) -> ("error out"=w484:errorcluster, "VISA resource name out"=w483:refnum<visa-resource-name>)  [unwired: 4 in, 1 out]
              }
              frame True {
              }
            }
          }
        }
        n217 = flat-sequence {
          tunnel: w376 -> [w504]
          tunnel: w348 -> [w505]
          tunnel: [w501] -> w375
          tunnel: [w511] -> w373
          tunnel: [w490] -> w371
          tunnel: [w492] -> w369
          tunnel: w344 -> [w491]
          tunnel: w343 -> [w488]
          tunnel: w328 -> [w489]
          tunnel: [w487] -> w317
          tunnel: w375 -> [w530]
          tunnel: [w530] -> w374
          tunnel: w373 -> [w529]
          tunnel: [w529] -> w372
          tunnel: w371 -> [w528]
          tunnel: [w526] -> w370
          tunnel: w369 -> [w527]
          tunnel: [w527] -> w368
          tunnel: w374 -> [w533]
          tunnel: w372 -> [w534]
          tunnel: w370 -> [w532]
          tunnel: w368 -> [w531]
          tunnel: [w531] -> w325
          frame #0 {
            w510 = 0.5 ("Delay Time (s)")
            n218 = call "Applied Send Command.vi"("error in (no error)"=w504, "Command"=T1."Immediate Position?", "VISA resource name"=w505) -> ("error out"=w507:errorcluster, "read buffer"=w508:string, "VISA resource name out"=w502:refnum<visa-resource-name>)  [unwired: 4 in]
            n219 = To Long Integer(number=w491) -> (32bit integer=w522:i32)
            n220 = To Long Integer(number=w488) -> (32bit integer=w523:i32)
            n221 = Hexadecimal String To Number(string=w508, offset=3) -> (number=w512:u32)  [unwired: 1 in, 1 out]
            n222 = To Long Integer(number=w512) -> (32bit integer=w513:i32)
            n223 = property on="Y steps/rev" class="DigNum (strict)"() -> ("Value"=w519:u32)  [unwired: 2 in, 2 out]
            n224 = property on="Y Step PV" class="DigNum (strict)"("Val(Sgnl)"=w513) -> ()  [unwired: 2 in, 2 out]
            n225 = In Range and Coerce(upper limit=w522, x=w513, lower limit=w523) -> (In Range?=w521:bool)  [unwired: 1 out]
            n226 = To Double Precision Float(number=w513) -> (double precision float=w514:dbl)
            n227 = To Double Precision Float(number=w519) -> (double precision float=w520:dbl)
            n228 = Divide(x=w514, y=w520) -> (x/y=w518:dbl)
            n229 = And(x=w521, y=w489) -> (x .and. y?=w490:bool)
            n230 = property on="Y in Range" class="Bool (strict)"("Val(Sgnl)"=w490) -> ()  [unwired: 2 in, 2 out]
            n231 = call "Time Delay4"("error in (no error)"=w507, "Delay Time (s)"=w510) -> ("error out"=w500:errorcluster)  [unwired: 9 in]
            n232 = property on="Y mm/rev" class="DigNum (strict)"() -> ("Value"=w517:dbl)  [unwired: 2 in, 2 out]
            n233 = property on="Y offset mm" class="DigNum (strict)"() -> ("Value"=w515:dbl)  [unwired: 2 in, 2 out]
            n234 = Multiply(x=w518, y=w517) -> (x*y=w516:dbl)
            n235 = call "Applied Send Command.vi"("error in (no error)"=w500, "Command"=T1."Request Status", "VISA resource name"=w502) -> ("error out"=w499:errorcluster, "read buffer"=w496:string, "VISA resource name out"=w501:refnum<visa-resource-name>)  [unwired: 4 in]
            n236 = call "Time Delay3"("error in (no error)"=w499, "Delay Time (s)"=w510) -> ("error out"=w511:errorcluster)  [unwired: 9 in]
            n237 = Add(x=w516, y=w515) -> (x+y=w487:dbl)
            n238 = String Subset(string=w496, offset (0)=0, length (rest)=1 ("length (rest)")) -> (substring=w494:string)
            n239 = property on="Y Position mm PV" class="DigNum (strict)"("Val(Sgnl)"=w487) -> ()  [unwired: 2 in, 2 out]
            n240 = Equal?(x=w494, y="R") -> (x = y?=w509:bool)
            n241 = Not Equal?(x=w494, y="R") -> (x != y?=w492:bool)
            n242 = property on="Y Ready" class="Bool (strict)"("Val(Sgnl)"=w509) -> ()  [unwired: 2 in, 2 out]
            n243 = property on="Y in Motion" class="Bool (strict)"("Val(Sgnl)"=w492) -> ()  [unwired: 2 in, 2 out]
          }
          frame #1 {
            n244 = local read "NC"() -> (w525:bool)
            n245 = Or(x=w528, y=w525) -> (x .or. y?=w526:bool)
          }
          frame #2 {
            n246 = case shown="False" w532 {
              tunnel: w533 -> [w536 w541]
              tunnel: [w538 w541] -> _
              tunnel: [w537 w540] -> _
              tunnel: w534 -> [w535 w540]
              frame False {
                n247 = call "Applied Send Command.vi"("error in (no error)"=w535, "Command"=T1."Stop & Kill Buffer", "VISA resource name"=w536) -> ("error out"=w537:errorcluster, "VISA resource name out"=w538:refnum<visa-resource-name>)  [unwired: 4 in, 1 out]
              }
              frame True {
              }
            }
          }
        }
        n248 = Compound Arithmetic op=OR(w326, w325, w324) -> (w327:bool)
        n249 = case shown="False" w327 {
          tunnel: [T2."Enabled" ("Disabled") T2."Disabled and Grayed Out" ("Disabled")] -> w323
          frame False {
          }
          frame True {
          }
        }
        n250 = Build Array("APX:PiezoX", "APX:PiezoY", "APX:PiezoZ") -> (w322:string[])
        n251 = Build Array(w318, w317, w316) -> (w315:dbl[])
        n252 = call-poly <userlib>:"CaLabPut.vi"("Values"=w315, "PV Names"=w322) -> ()  [unwired: 6 in, 4 out]
        n253 = property on="Jog X-" class="Bool"("DisabledEnum"=w323) -> ()  [unwired: 2 in, 2 out]
        n254 = property on="Jog X+" class="Bool"("DisabledEnum"=w323) -> ()  [unwired: 2 in, 2 out]
        n255 = property on="Jog Y+" class="Bool"("DisabledEnum"=w323) -> ()  [unwired: 2 in, 2 out]
        n256 = property on="Jog Z+" class="Bool"("DisabledEnum"=w323) -> ()  [unwired: 2 in, 2 out]
        n257 = property on="Jog Y-" class="Bool"("DisabledEnum"=w323) -> ()  [unwired: 2 in, 2 out]
        n258 = property on="Jog Z-" class="Bool"("DisabledEnum"=w323) -> ()  [unwired: 2 in, 2 out]
      }
      event "Reset Y Position mm", "Reset X Position mm", "Reset Z Position mm": Value Change {
        n259 = event-data() -> ()  [unwired: 1 in, 5 out]
        n260 = property on="Reset Y Position mm" class="DigNum (strict)"() -> ("Value"=w568:dbl)  [unwired: 2 in, 2 out]
        n261 = property on="Reset X Position mm" class="DigNum (strict)"() -> ("Value"=w559:dbl)  [unwired: 2 in, 2 out]
        n262 = property on="Reset Z Position mm" class="DigNum (strict)"() -> ("Value"=w550:dbl)  [unwired: 2 in, 2 out]
        n263 = property on="Y offset mm" class="DigNum (strict)"() -> ("Value"=w560:dbl)  [unwired: 2 in, 2 out]
        n264 = property on="X offset mm" class="DigNum (strict)"() -> ("Value"=w551:dbl)  [unwired: 2 in, 2 out]
        n265 = property on="Z offset mm" class="DigNum (strict)"() -> ("Value"=w542:dbl)  [unwired: 2 in, 2 out]
        n266 = Subtract(x=w568, y=w560) -> (x-y=w567:dbl)
        n267 = Subtract(x=w559, y=w551) -> (x-y=w558:dbl)
        n268 = Subtract(x=w550, y=w542) -> (x-y=w549:dbl)
        n269 = property on="Y steps/rev" class="DigNum (strict)"() -> ("Value"=w562:u32)  [unwired: 2 in, 2 out]
        n270 = property on="X steps/rev" class="DigNum (strict)"() -> ("Value"=w553:u32)  [unwired: 2 in, 2 out]
        n271 = property on="Z steps/rev" class="DigNum (strict)"() -> ("Value"=w544:u32)  [unwired: 2 in, 2 out]
        n272 = property on="Y mm/rev" class="DigNum (strict)"() -> ("Value"=w561:dbl)  [unwired: 2 in, 2 out]
        n273 = property on="X mm/rev" class="DigNum (strict)"() -> ("Value"=w552:dbl)  [unwired: 2 in, 2 out]
        n274 = property on="Z mm/rev" class="DigNum (strict)"() -> ("Value"=w543:dbl)  [unwired: 2 in, 2 out]
        n275 = Divide(x=w567, y=w561) -> (x/y=w566:dbl)
        n276 = Divide(x=w558, y=w552) -> (x/y=w557:dbl)
        n277 = Divide(x=w549, y=w543) -> (x/y=w548:dbl)
        n278 = To Double Precision Float(number=w562) -> (double precision float=w565:dbl)
        n279 = To Double Precision Float(number=w553) -> (double precision float=w556:dbl)
        n280 = To Double Precision Float(number=w544) -> (double precision float=w547:dbl)
        n281 = Multiply(x=w566, y=w565) -> (x*y=w564:dbl)
        n282 = Multiply(x=w557, y=w556) -> (x*y=w555:dbl)
        n283 = Multiply(x=w548, y=w547) -> (x*y=w546:dbl)
        n284 = To Long Integer(number=w564) -> (32bit integer=w563:i32)
        n285 = To Long Integer(number=w555) -> (32bit integer=w554:i32)
        n286 = To Long Integer(number=w546) -> (32bit integer=w545:i32)
        n287 = property on="Reset Y Motor Steps" class="DigNum (strict)"("Val(Sgnl)"=w563) -> ()  [unwired: 2 in, 2 out]
        n288 = property on="Reset X Motor Steps" class="DigNum (strict)"("Val(Sgnl)"=w554) -> ()  [unwired: 2 in, 2 out]
        n289 = property on="Reset Z Motor Steps" class="DigNum (strict)"("Val(Sgnl)"=w545) -> ()  [unwired: 2 in, 2 out]
      }
      event "Y Velocity SP step/sec", "X Velocity SP step/sec", "Z Velocity SP step/sec", "Y Step SP", "X Step SP", "Z Step SP": Value Change {
        n290 = event-data() -> ()  [unwired: 1 in, 5 out]
        n291 = property on="X Velocity SP step/sec" class="DigNum (strict)"() -> ("Value"=w604:i32)  [unwired: 2 in, 2 out]
        n292 = property on="Y Velocity SP step/sec" class="DigNum (strict)"() -> ("Value"=w610:i32)  [unwired: 2 in, 2 out]
        n293 = property on="Z Velocity SP step/sec" class="DigNum (strict)"() -> ("Value"=w598:i32)  [unwired: 2 in, 2 out]
        n294 = property on="X steps/rev" class="DigNum (strict)"() -> ("Value"=w581:u32)  [unwired: 2 in, 2 out]
        n295 = property on="X steps/rev" class="DigNum (strict)"() -> ("Value"=w602:u32)  [unwired: 2 in, 2 out]
        n296 = property on="Y steps/rev" class="DigNum (strict)"() -> ("Value"=w589:u32)  [unwired: 2 in, 2 out]
        n297 = property on="Y steps/rev" class="DigNum (strict)"() -> ("Value"=w608:u32)  [unwired: 2 in, 2 out]
        n298 = property on="Z steps/rev" class="DigNum (strict)"() -> ("Value"=w573:u32)  [unwired: 2 in, 2 out]
        n299 = property on="Z steps/rev" class="DigNum (strict)"() -> ("Value"=w596:u32)  [unwired: 2 in, 2 out]
        n300 = property on="X Step SP" class="DigNum (strict)"() -> ("Value"=w583:i32)  [unwired: 2 in, 2 out]
        n301 = property on="Y Step SP" class="DigNum (strict)"() -> ("Value"=w591:i32)  [unwired: 2 in, 2 out]
        n302 = property on="Z Step SP" class="DigNum (strict)"() -> ("Value"=w575:i32)  [unwired: 2 in, 2 out]
        n303 = To Double Precision Float(number=w583) -> (double precision float=w584:dbl)
        n304 = To Double Precision Float(number=w581) -> (double precision float=w587:dbl)
        n305 = To Double Precision Float(number=w604) -> (double precision float=w605:dbl)
        n306 = To Double Precision Float(number=w602) -> (double precision float=w607:dbl)
        n307 = To Double Precision Float(number=w591) -> (double precision float=w592:dbl)
        n308 = To Double Precision Float(number=w589) -> (double precision float=w595:dbl)
        n309 = To Double Precision Float(number=w610) -> (double precision float=w611:dbl)
        n310 = To Double Precision Float(number=w608) -> (double precision float=w613:dbl)
        n311 = To Double Precision Float(number=w575) -> (double precision float=w576:dbl)
        n312 = To Double Precision Float(number=w573) -> (double precision float=w579:dbl)
        n313 = To Double Precision Float(number=w598) -> (double precision float=w599:dbl)
        n314 = To Double Precision Float(number=w596) -> (double precision float=w601:dbl)
        n315 = property on="X mm/rev" class="DigNum (strict)"() -> ("Value"=w570:dbl)  [unwired: 2 in, 2 out]
        n316 = property on="Y mm/rev" class="DigNum (strict)"() -> ("Value"=w569:dbl)  [unwired: 2 in, 2 out]
        n317 = property on="Z mm/rev" class="DigNum (strict)"() -> ("Value"=w571:dbl)  [unwired: 2 in, 2 out]
        n318 = Divide(x=w584, y=w587) -> (x/y=w586:dbl)
        n319 = Divide(x=w605, y=w607) -> (x/y=w606:dbl)
        n320 = Divide(x=w592, y=w595) -> (x/y=w594:dbl)
        n321 = Divide(x=w611, y=w613) -> (x/y=w612:dbl)
        n322 = Divide(x=w576, y=w579) -> (x/y=w578:dbl)
        n323 = Divide(x=w599, y=w601) -> (x/y=w600:dbl)
        n324 = property on="X offset mm" class="DigNum (strict)"() -> ("Value"=w580:dbl)  [unwired: 2 in, 2 out]
        n325 = property on="Y offset mm" class="DigNum (strict)"() -> ("Value"=w588:dbl)  [unwired: 2 in, 2 out]
        n326 = property on="Z offset mm" class="DigNum (strict)"() -> ("Value"=w572:dbl)  [unwired: 2 in, 2 out]
        n327 = Multiply(x=w586, y=w570) -> (x*y=w585:dbl)
        n328 = Multiply(x=w606, y=w570) -> (x*y=w603:dbl)
        n329 = Multiply(x=w594, y=w569) -> (x*y=w593:dbl)
        n330 = Multiply(x=w612, y=w569) -> (x*y=w609:dbl)
        n331 = Multiply(x=w578, y=w571) -> (x*y=w577:dbl)
        n332 = Multiply(x=w600, y=w571) -> (x*y=w597:dbl)
        n333 = property on="X Velocity MV mm/sec" class="DigNum (strict)"("Val(Sgnl)"=w603) -> ()  [unwired: 2 in, 2 out]
        n334 = property on="Y Velocity MV mm/sec" class="DigNum (strict)"("Val(Sgnl)"=w609) -> ()  [unwired: 2 in, 2 out]
        n335 = property on="Z Velocity MV mm/sec" class="DigNum (strict)"("Val(Sgnl)"=w597) -> ()  [unwired: 2 in, 2 out]
        n336 = Add(x=w585, y=w580) -> (x+y=w582:dbl)
        n337 = Add(x=w593, y=w588) -> (x+y=w590:dbl)
        n338 = Add(x=w577, y=w572) -> (x+y=w574:dbl)
        n339 = property on="X Position MV mm" class="DigNum (strict)"("Val(Sgnl)"=w582) -> ()  [unwired: 2 in, 2 out]
        n340 = property on="Y Position MV mm" class="DigNum (strict)"("Val(Sgnl)"=w590) -> ()  [unwired: 2 in, 2 out]
        n341 = property on="Z Position MV mm" class="DigNum (strict)"("Val(Sgnl)"=w574) -> ()  [unwired: 2 in, 2 out]
      }
      event "Y Jog Set": Mouse Down {
        n342 = event-data() -> ()  [unwired: 1 in, 7 out]
        n343 = property on="Y offset mm" class="DigNum (strict)"() -> ("Value"=w628:dbl)  [unwired: 2 in, 2 out]
        n344 = property on="APX:FYstep" class="DigNum (strict)"() -> ("Value"=w627:dbl)  [unwired: 2 in, 2 out]
        n345 = property on="FY Velocity SP mm/sec" class="DigNum (strict)"() -> ("Value"=w621:dbl)  [unwired: 2 in, 2 out]
        n346 = property on="Y steps/rev" class="DigNum (strict)"() -> ("Value"=w630:u32)  [unwired: 2 in, 2 out]
        n347 = property on="Y mm/rev" class="DigNum (strict)"() -> ("Value"=w614:dbl)  [unwired: 2 in, 2 out]
        n348 = Subtract(x=w627, y=w628) -> (x-y=w631:dbl)
        n349 = Divide(x=w621, y=w614) -> (x/y=w622:dbl)
        n350 = Divide(x=w631, y=w614) -> (x/y=w632:dbl)
        n351 = To Double Precision Float(number=w630) -> (double precision float=w615:dbl)
        n352 = property on="Y Velocity SP step/sec" class="DigNum (strict)"() -> ("Maximum"=w617:dbl)  [unwired: 2 in, 2 out]
        n353 = property on="Y Velocity SP step/sec" class="DigNum (strict)"() -> ("Minimum"=w616:dbl)  [unwired: 2 in, 2 out]
        n354 = property on="Y Step SP" class="DigNum (strict)"() -> ("Maximum"=w624:dbl)  [unwired: 2 in, 2 out]
        n355 = property on="Y Step SP" class="DigNum (strict)"() -> ("Minimum"=w623:dbl)  [unwired: 2 in, 2 out]
        n356 = Multiply(x=w622, y=w615) -> (x*y=w619:dbl)
        n357 = Multiply(x=w632, y=w615) -> (x*y=w626:dbl)
        n358 = In Range and Coerce(upper limit=w617, x=w619, lower limit=w616) -> (coerced(x)=w618:dbl)  [unwired: 1 out]
        n359 = In Range and Coerce(upper limit=w624, x=w626, lower limit=w623) -> (coerced(x)=w625:dbl)  [unwired: 1 out]
        n360 = To Long Integer(number=w618) -> (32bit integer=w620:i32)
        n361 = To Long Integer(number=w625) -> (32bit integer=w629:i32)
        n362 = property on="Y Velocity SP step/sec" class="DigNum (strict)"("Val(Sgnl)"=w620) -> ()  [unwired: 2 in, 2 out]
        n363 = property on="Y Step SP" class="DigNum (strict)"("Val(Sgnl)"=w629) -> ()  [unwired: 2 in, 2 out]
      }
      event "X Jog Set": Mouse Down {
        n364 = event-data() -> ()  [unwired: 1 in, 7 out]
        n365 = property on="X offset mm" class="DigNum (strict)"() -> ("Value"=w647:dbl)  [unwired: 2 in, 2 out]
        n366 = property on="APX:FXstep" class="DigNum (strict)"() -> ("Value"=w646:dbl)  [unwired: 2 in, 2 out]
        n367 = property on="FX Velocity SP mm/sec" class="DigNum (strict)"() -> ("Value"=w640:dbl)  [unwired: 2 in, 2 out]
        n368 = property on="X steps/rev" class="DigNum (strict)"() -> ("Value"=w649:u32)  [unwired: 2 in, 2 out]
        n369 = property on="X mm/rev" class="DigNum (strict)"() -> ("Value"=w633:dbl)  [unwired: 2 in, 2 out]
        n370 = Subtract(x=w646, y=w647) -> (x-y=w650:dbl)
        n371 = Divide(x=w640, y=w633) -> (x/y=w641:dbl)
        n372 = Divide(x=w650, y=w633) -> (x/y=w651:dbl)
        n373 = To Double Precision Float(number=w649) -> (double precision float=w634:dbl)
        n374 = property on="X Velocity SP step/sec" class="DigNum (strict)"() -> ("Maximum"=w636:dbl)  [unwired: 2 in, 2 out]
        n375 = property on="X Velocity SP step/sec" class="DigNum (strict)"() -> ("Minimum"=w635:dbl)  [unwired: 2 in, 2 out]
        n376 = property on="X Step SP" class="DigNum (strict)"() -> ("Maximum"=w643:dbl)  [unwired: 2 in, 2 out]
        n377 = property on="X Step SP" class="DigNum (strict)"() -> ("Minimum"=w642:dbl)  [unwired: 2 in, 2 out]
        n378 = Multiply(x=w641, y=w634) -> (x*y=w638:dbl)
        n379 = Multiply(x=w651, y=w634) -> (x*y=w645:dbl)
        n380 = In Range and Coerce(upper limit=w636, x=w638, lower limit=w635) -> (coerced(x)=w637:dbl)  [unwired: 1 out]
        n381 = In Range and Coerce(upper limit=w643, x=w645, lower limit=w642) -> (coerced(x)=w644:dbl)  [unwired: 1 out]
        n382 = To Long Integer(number=w637) -> (32bit integer=w639:i32)
        n383 = To Long Integer(number=w644) -> (32bit integer=w648:i32)
        n384 = property on="X Velocity SP step/sec" class="DigNum (strict)"("Val(Sgnl)"=w639) -> ()  [unwired: 2 in, 2 out]
        n385 = property on="X Step SP" class="DigNum (strict)"("Val(Sgnl)"=w648) -> ()  [unwired: 2 in, 2 out]
      }
      event "Z Jog Set": Mouse Down {
        n386 = event-data() -> ()  [unwired: 1 in, 7 out]
        n387 = property on="Z offset mm" class="DigNum (strict)"() -> ("Value"=w655:dbl)  [unwired: 2 in, 2 out]
        n388 = property on="APX:FZabs" class="DigNum (strict)"() -> ("Value"=w653:dbl)  [unwired: 2 in, 2 out]
        n389 = property on="FZ Velocity SP mm/sec" class="DigNum (strict)"() -> ("Value"=w668:dbl)  [unwired: 2 in, 2 out]
        n390 = property on="APX:Fzstep" class="DigNum (strict)"() -> ("Value"=w674:dbl)  [unwired: 2 in, 2 out]
        n391 = property on="Z steps/rev" class="DigNum (strict)"() -> ("Value"=w676:u32)  [unwired: 2 in, 2 out]
        n392 = property on="Z mm/rev" class="DigNum (strict)"() -> ("Value"=w656:dbl)  [unwired: 2 in, 2 out]
        n393 = Subtract(x=w653, y=w655) -> (x-y=w654:dbl)
        n394 = Divide(x=w674, y=w656) -> (x/y=w677:dbl)
        n395 = Divide(x=w668, y=w656) -> (x/y=w669:dbl)
        n396 = Divide(x=w654, y=w656) -> (x/y=w657:dbl)
        n397 = property on="Z Velocity SP step/sec" class="DigNum (strict)"() -> ("Maximum"=w664:dbl)  [unwired: 2 in, 2 out]
        n398 = property on="Z Velocity SP step/sec" class="DigNum (strict)"() -> ("Minimum"=w663:dbl)  [unwired: 2 in, 2 out]
        n399 = To Double Precision Float(number=w676) -> (double precision float=w658:dbl)
        n400 = property on="Z Step SP" class="DigNum (strict)"() -> ("Maximum"=w671:dbl)  [unwired: 2 in, 2 out]
        n401 = property on="Z Step SP" class="DigNum (strict)"() -> ("Minimum"=w670:dbl)  [unwired: 2 in, 2 out]
        n402 = property on="Z Step SP" class="DigNum (strict)"() -> ("Maximum"=w661:dbl)  [unwired: 2 in, 2 out]
        n403 = property on="Z Step SP" class="DigNum (strict)"() -> ("Minimum"=w660:dbl)  [unwired: 2 in, 2 out]
        n404 = Multiply(x=w677, y=w658) -> (x*y=w673:dbl)
        n405 = Multiply(x=w669, y=w658) -> (x*y=w666:dbl)
        n406 = Multiply(x=w657, y=w658) -> (x*y=w659:dbl)
        n407 = In Range and Coerce(upper limit=w671, x=w673, lower limit=w670) -> (coerced(x)=w672:dbl)  [unwired: 1 out]
        n408 = In Range and Coerce(upper limit=w664, x=w666, lower limit=w663) -> (coerced(x)=w665:dbl)  [unwired: 1 out]
        n409 = In Range and Coerce(upper limit=w661, x=w659, lower limit=w660) -> (coerced(x)=w662:dbl)  [unwired: 1 out]
        n410 = To Long Integer(number=w672) -> (32bit integer=w675:i32)
        n411 = To Long Integer(number=w665) -> (32bit integer=w667:i32)
        n412 = To Long Integer(number=w662) -> (32bit integer=w652:i32)
        n413 = property on="Z Step SP" class="DigNum (strict)"("Val(Sgnl)"=w675) -> ()  [unwired: 2 in, 2 out]
        n414 = property on="Z Velocity SP step/sec" class="DigNum (strict)"("Val(Sgnl)"=w667) -> ()  [unwired: 2 in, 2 out]
        n415 = property on="Z Abso SP" class="DigNum (strict)"("Val(Sgnl)"=w652) -> ()  [unwired: 2 in, 2 out]
      }
      event "Jog Y+": Mouse Up {
        n416 = event-data() -> ()  [unwired: 1 in, 7 out]
        n417 = flat-sequence {
          tunnel: [w694] -> w683
          tunnel: [w689] -> w682
          tunnel: [w688] -> w679
          tunnel: w680 -> [w693]
          tunnel: w681 -> [w692]
          tunnel: [w705] -> w685
          tunnel: [w700] -> w684
          tunnel: w683 -> [w703]
          tunnel: w682 -> [w704]
          tunnel: w679 -> [w701]
          tunnel: [w701] -> w678
          tunnel: [w710] -> w686
          tunnel: [w713] -> w687
          tunnel: w685 -> [w712]
          tunnel: w684 -> [w711]
          tunnel: w678 -> [w714]
          frame #0 {
            w688 = 0.5 ("Delay Time (s)")
            # "Velocity Setting"
            n418 = property on="Y Velocity SP step/sec" class="DigNum (strict)"() -> ("Value"=w697:i32)  [unwired: 2 in, 2 out]
            n419 = property on="Y steps/rev" class="DigNum (strict)"() -> ("Value"=w696:u32)  [unwired: 2 in, 2 out]
            n420 = Number To Decimal String(number=w697) -> ()  [unwired: 1 in, 1 out]
            n421 = Divide(x=w697, y=w696) -> (x/y=w698:dbl)
            n422 = Number To Fractional String(number=w698) -> (F-format string=w691:string)  [unwired: 3 in]
            n423 = call "Applied Send Command.vi"("error in (no error)"=w693, "Extra"=w691, "Command"=T1."Velocity Setting", "VISA resource name"=w692) -> ("error out"=w690:errorcluster, "VISA resource name out"=w694:refnum<visa-resource-name>)  [unwired: 3 in, 1 out]
            n424 = call "Time Delay22"("error in (no error)"=w690, "Delay Time (s)"=w688) -> ("error out"=w689:errorcluster)  [unwired: 9 in]
          }
          frame #1 {
            # "Move to Abs Position"
            n425 = property on="Y Step SP" class="DigNum (strict)"() -> ("Value"=w707:i32)  [unwired: 2 in, 2 out]
            n426 = Number To Decimal String(number=w707) -> (decimal integer string=w702:string)  [unwired: 1 in]
            n427 = call "Applied Send Command.vi"("error in (no error)"=w704, "Extra"=w702, "Command"=T1."Distance or Position", "VISA resource name"=w703) -> ("error out"=w699:errorcluster, "VISA resource name out"=w705:refnum<visa-resource-name>)  [unwired: 3 in, 1 out]
            n428 = call "Time Delay"("error in (no error)"=w699, "Delay Time (s)"=w701) -> ("error out"=w700:errorcluster)  [unwired: 9 in]
          }
          frame #2 {
            n429 = call "Applied Send Command.vi"("error in (no error)"=w711, "Command"=T1."Feed to Length", "VISA resource name"=w712) -> ("error out"=w708:errorcluster, "VISA resource name out"=w713:refnum<visa-resource-name>)  [unwired: 4 in, 1 out]
            n430 = call "Time Delay23"("error in (no error)"=w708, "Delay Time (s)"=w714) -> ("error out"=w710:errorcluster)  [unwired: 9 in]
          }
        }
      }
      event "Jog Y-": Mouse Up {
        n431 = event-data() -> ()  [unwired: 1 in, 8 out]
        n432 = flat-sequence {
          tunnel: [w731] -> w720
          tunnel: [w726] -> w719
          tunnel: [w725] -> w716
          tunnel: w717 -> [w730]
          tunnel: w718 -> [w729]
          tunnel: [w744] -> w722
          tunnel: [w739] -> w721
          tunnel: w720 -> [w742]
          tunnel: w719 -> [w743]
          tunnel: w716 -> [w740]
          tunnel: [w740] -> w715
          tunnel: [w749] -> w723
          tunnel: [w752] -> w724
          tunnel: w722 -> [w751]
          tunnel: w721 -> [w750]
          tunnel: w715 -> [w753]
          frame #0 {
            w725 = 0.5 ("Delay Time (s)")
            # "Velocity Setting"
            n433 = property on="Y Velocity SP step/sec" class="DigNum (strict)"() -> ("Value"=w734:i32)  [unwired: 2 in, 2 out]
            n434 = property on="Y steps/rev" class="DigNum (strict)"() -> ("Value"=w733:u32)  [unwired: 2 in, 2 out]
            n435 = Number To Decimal String(number=w734) -> ()  [unwired: 1 in, 1 out]
            n436 = Divide(x=w734, y=w733) -> (x/y=w735:dbl)
            n437 = Number To Fractional String(number=w735) -> (F-format string=w728:string)  [unwired: 3 in]
            n438 = call "Applied Send Command.vi"("error in (no error)"=w730, "Extra"=w728, "Command"=T1."Velocity Setting", "VISA resource name"=w729) -> ("error out"=w727:errorcluster, "VISA resource name out"=w731:refnum<visa-resource-name>)  [unwired: 3 in, 1 out]
            n439 = call "Time Delay18"("error in (no error)"=w727, "Delay Time (s)"=w725) -> ("error out"=w726:errorcluster)  [unwired: 9 in]
          }
          frame #1 {
            # "Move to Abs Position"
            n440 = property on="Y Step SP" class="DigNum (strict)"() -> ("Value"=w746:i32)  [unwired: 2 in, 2 out]
            n441 = Multiply(x=-1, y=w746) -> (x*y=w737:i32)
            n442 = Number To Decimal String(number=w737) -> (decimal integer string=w741:string)  [unwired: 1 in]
            n443 = call "Applied Send Command.vi"("error in (no error)"=w743, "Extra"=w741, "Command"=T1."Distance or Position", "VISA resource name"=w742) -> ("error out"=w738:errorcluster, "VISA resource name out"=w744:refnum<visa-resource-name>)  [unwired: 3 in, 1 out]
            n444 = call "Time Delay10"("error in (no error)"=w738, "Delay Time (s)"=w740) -> ("error out"=w739:errorcluster)  [unwired: 9 in]
          }
          frame #2 {
            n445 = call "Applied Send Command.vi"("error in (no error)"=w750, "Command"=T1."Feed to Length", "VISA resource name"=w751) -> ("error out"=w747:errorcluster, "VISA resource name out"=w752:refnum<visa-resource-name>)  [unwired: 4 in, 1 out]
            n446 = call "Time Delay9"("error in (no error)"=w747, "Delay Time (s)"=w753) -> ("error out"=w749:errorcluster)  [unwired: 9 in]
          }
        }
      }
      event "Jog Z+": Mouse Up {
        n447 = event-data() -> ()  [unwired: 1 in, 7 out]
        n448 = flat-sequence {
          tunnel: [w767] -> w761
          tunnel: [w765] -> w760
          tunnel: [w764] -> w755
          tunnel: w758 -> [w768]
          tunnel: w759 -> [w769]
          tunnel: [w778] -> w763
          tunnel: [w777] -> w762
          tunnel: w761 -> [w779]
          tunnel: w760 -> [w781]
          tunnel: w755 -> [w775]
          tunnel: [w775] -> w754
          tunnel: [w790] -> w757
          tunnel: [w787] -> w756
          tunnel: w763 -> [w788]
          tunnel: w762 -> [w786]
          tunnel: w754 -> [w789]
          frame #0 {
            w764 = 0.1 ("Delay Time (s)")
            n449 = property on="Z Velocity SP step/sec" class="DigNum (strict)"() -> ("Value"=w771:i32)  [unwired: 2 in, 2 out]
            n450 = property on="Z steps/rev" class="DigNum (strict)"() -> ("Value"=w770:u32)  [unwired: 2 in, 2 out]
            n451 = Divide(x=w771, y=w770) -> (x/y=w772:dbl)
            n452 = Number To Fractional String(number=w772) -> (F-format string=w773:string)  [unwired: 3 in]
            n453 = call "Applied Send Command.vi"("error in (no error)"=w768, "Extra"=w773, "Command"=T1."Velocity Setting", "VISA resource name"=w769) -> ("error out"=w766:errorcluster, "VISA resource name out"=w767:refnum<visa-resource-name>)  [unwired: 3 in, 1 out]
            n454 = call "Time Delay52"("error in (no error)"=w766, "Delay Time (s)"=w764) -> ("error out"=w765:errorcluster)  [unwired: 9 in]
          }
          frame #1 {
            # "Move to Abs Position"
            n455 = property on="Z Step SP" class="DigNum (strict)"() -> ("Value"=w783:i32)  [unwired: 2 in, 2 out]
            n456 = Number To Decimal String(number=w783) -> (decimal integer string=w780:string)  [unwired: 1 in]
            n457 = call "Applied Send Command.vi"("error in (no error)"=w781, "Extra"=w780, "Command"=T1."Distance or Position", "VISA resource name"=w779) -> ("error out"=w776:errorcluster, "VISA resource name out"=w778:refnum<visa-resource-name>)  [unwired: 3 in, 1 out]
            n458 = call "Time Delay51"("error in (no error)"=w776, "Delay Time (s)"=w775) -> ("error out"=w777:errorcluster)  [unwired: 9 in]
          }
          frame #2 {
            n459 = call "Applied Send Command.vi"("error in (no error)"=w786, "Command"=T1."Feed to Length", "VISA resource name"=w788) -> ("error out"=w784:errorcluster, "VISA resource name out"=w787:refnum<visa-resource-name>)  [unwired: 4 in, 1 out]
            n460 = call "Time Delay28"("error in (no error)"=w784, "Delay Time (s)"=w789) -> ("error out"=w790:errorcluster)  [unwired: 9 in]
          }
        }
      }
      event "Move Z": Mouse Up {
        n461 = event-data() -> ()  [unwired: 1 in, 7 out]
        n462 = flat-sequence {
          tunnel: [w804] -> w798
          tunnel: [w802] -> w797
          tunnel: [w801] -> w792
          tunnel: w795 -> [w805]
          tunnel: w796 -> [w806]
          tunnel: [w815] -> w800
          tunnel: [w814] -> w799
          tunnel: w798 -> [w816]
          tunnel: w797 -> [w818]
          tunnel: w792 -> [w812]
          tunnel: [w812] -> w791
          tunnel: [w827] -> w794
          tunnel: [w824] -> w793
          tunnel: w800 -> [w825]
          tunnel: w799 -> [w823]
          tunnel: w791 -> [w826]
          frame #0 {
            w801 = 0.1 ("Delay Time (s)")
            n463 = property on="Z Velocity SP step/sec" class="DigNum (strict)"() -> ("Value"=w808:i32)  [unwired: 2 in, 2 out]
            n464 = property on="Z steps/rev" class="DigNum (strict)"() -> ("Value"=w807:u32)  [unwired: 2 in, 2 out]
            n465 = Divide(x=w808, y=w807) -> (x/y=w809:dbl)
            n466 = Number To Fractional String(number=w809) -> (F-format string=w810:string)  [unwired: 3 in]
            n467 = call "Applied Send Command.vi"("error in (no error)"=w805, "Extra"=w810, "Command"=T1."Velocity Setting", "VISA resource name"=w806) -> ("error out"=w803:errorcluster, "VISA resource name out"=w804:refnum<visa-resource-name>)  [unwired: 3 in, 1 out]
            n468 = call "Time Delay26"("error in (no error)"=w803, "Delay Time (s)"=w801) -> ("error out"=w802:errorcluster)  [unwired: 9 in]
          }
          frame #1 {
            # "Move to Abs Position"
            n469 = property on="Z Abso SP" class="DigNum (strict)"() -> ("Value"=w820:i32)  [unwired: 2 in, 2 out]
            n470 = Number To Decimal String(number=w820) -> (decimal integer string=w817:string)  [unwired: 1 in]
            n471 = call "Applied Send Command.vi"("error in (no error)"=w818, "Extra"=w817, "Command"=T1."Distance or Position", "VISA resource name"=w816) -> ("error out"=w813:errorcluster, "VISA resource name out"=w815:refnum<visa-resource-name>)  [unwired: 3 in, 1 out]
            n472 = call "Time Delay25"("error in (no error)"=w813, "Delay Time (s)"=w812) -> ("error out"=w814:errorcluster)  [unwired: 9 in]
          }
          frame #2 {
            n473 = call "Applied Send Command.vi"("error in (no error)"=w823, "Command"=T1."Feed to Position", "VISA resource name"=w825) -> ("error out"=w821:errorcluster, "VISA resource name out"=w824:refnum<visa-resource-name>)  [unwired: 4 in, 1 out]
            n474 = call "Time Delay24"("error in (no error)"=w821, "Delay Time (s)"=w826) -> ("error out"=w827:errorcluster)  [unwired: 9 in]
          }
        }
      }
      event "Jog Z-": Mouse Up {
        n475 = event-data() -> ()  [unwired: 1 in, 8 out]
        n476 = flat-sequence {
          tunnel: [w841] -> w835
          tunnel: [w839] -> w834
          tunnel: [w838] -> w829
          tunnel: w832 -> [w842]
          tunnel: w833 -> [w843]
          tunnel: [w854] -> w837
          tunnel: [w853] -> w836
          tunnel: w835 -> [w855]
          tunnel: w834 -> [w857]
          tunnel: w829 -> [w851]
          tunnel: [w851] -> w828
          tunnel: [w866] -> w831
          tunnel: [w863] -> w830
          tunnel: w837 -> [w864]
          tunnel: w836 -> [w862]
          tunnel: w828 -> [w865]
          frame #0 {
            w838 = 0.1 ("Delay Time (s)")
            n477 = property on="Z Velocity SP step/sec" class="DigNum (strict)"() -> ("Value"=w845:i32)  [unwired: 2 in, 2 out]
            n478 = property on="Z steps/rev" class="DigNum (strict)"() -> ("Value"=w844:u32)  [unwired: 2 in, 2 out]
            n479 = Divide(x=w845, y=w844) -> (x/y=w846:dbl)
            n480 = Number To Fractional String(number=w846) -> (F-format string=w847:string)  [unwired: 3 in]
            n481 = call "Applied Send Command.vi"("error in (no error)"=w842, "Extra"=w847, "Command"=T1."Velocity Setting", "VISA resource name"=w843) -> ("error out"=w840:errorcluster, "VISA resource name out"=w841:refnum<visa-resource-name>)  [unwired: 3 in, 1 out]
            n482 = call "Time Delay21"("error in (no error)"=w840, "Delay Time (s)"=w838) -> ("error out"=w839:errorcluster)  [unwired: 9 in]
          }
          frame #1 {
            # "Move to Abs Position"
            n483 = property on="Z Step SP" class="DigNum (strict)"() -> ("Value"=w859:i32)  [unwired: 2 in, 2 out]
            n484 = Multiply(x=-1, y=w859) -> (x*y=w850:i32)
            n485 = Number To Decimal String(number=w850) -> (decimal integer string=w856:string)  [unwired: 1 in]
            n486 = call "Applied Send Command.vi"("error in (no error)"=w857, "Extra"=w856, "Command"=T1."Distance or Position", "VISA resource name"=w855) -> ("error out"=w852:errorcluster, "VISA resource name out"=w854:refnum<visa-resource-name>)  [unwired: 3 in, 1 out]
            n487 = call "Time Delay20"("error in (no error)"=w852, "Delay Time (s)"=w851) -> ("error out"=w853:errorcluster)  [unwired: 9 in]
          }
          frame #2 {
            n488 = call "Applied Send Command.vi"("error in (no error)"=w862, "Command"=T1."Feed to Length", "VISA resource name"=w864) -> ("error out"=w860:errorcluster, "VISA resource name out"=w863:refnum<visa-resource-name>)  [unwired: 4 in, 1 out]
            n489 = call "Time Delay19"("error in (no error)"=w860, "Delay Time (s)"=w865) -> ("error out"=w866:errorcluster)  [unwired: 9 in]
          }
        }
      }
      event "Jog X+": Mouse Up {
        n490 = event-data() -> ()  [unwired: 1 in, 7 out]
        n491 = flat-sequence {
          tunnel: [w881] -> w872
          tunnel: [w878] -> w870
          tunnel: [w877] -> w868
          tunnel: w876 -> [w883]
          tunnel: w875 -> [w882]
          tunnel: w872 -> [w890]
          tunnel: [w889] -> w871
          tunnel: w870 -> [w891]
          tunnel: [w892] -> w869
          tunnel: w868 -> [w888]
          tunnel: [w888] -> w867
          tunnel: w871 -> [w903]
          tunnel: w869 -> [w902]
          tunnel: [w901] -> w874
          tunnel: [w900] -> w873
          tunnel: w867 -> [w899]
          frame #0 {
            w877 = 0.1 ("Delay Time (s)")
            n492 = property on="X Velocity SP step/sec" class="DigNum (strict)"() -> ("Value"=w880:i32)  [unwired: 2 in, 2 out]
            n493 = property on="X steps/rev" class="DigNum (strict)"() -> ("Value"=w884:u32)  [unwired: 2 in, 2 out]
            n494 = Divide(x=w880, y=w884) -> (x/y=w885:dbl)
            n495 = Number To Fractional String(number=w885) -> (F-format string=w886:string)  [unwired: 3 in]
            n496 = call "Applied Send Command.vi"("error in (no error)"=w882, "Extra"=w886, "Command"=T1."Velocity Setting", "VISA resource name"=w883) -> ("error out"=w879:errorcluster, "VISA resource name out"=w881:refnum<visa-resource-name>)  [unwired: 3 in, 1 out]
            n497 = call "Time Delay14"("error in (no error)"=w879, "Delay Time (s)"=w877) -> ("error out"=w878:errorcluster)  [unwired: 9 in]
          }
          frame #1 {
            # "Distance/Position"
            n498 = property on="X Step SP" class="DigNum (strict)"() -> ("Value"=w893:i32)  [unwired: 2 in, 2 out]
            n499 = Number To Decimal String(number=w893) -> (decimal integer string=w895:string)  [unwired: 1 in]
            n500 = call "Applied Send Command.vi"("error in (no error)"=w891, "Extra"=w895, "Command"=T1."Distance or Position", "VISA resource name"=w890) -> ("error out"=w894:errorcluster, "VISA resource name out"=w889:refnum<visa-resource-name>)  [unwired: 3 in, 1 out]
            n501 = call "Time Delay31"("error in (no error)"=w894, "Delay Time (s)"=w888) -> ("error out"=w892:errorcluster)  [unwired: 9 in]
          }
          frame #2 {
            # "Feed to Position"
            n502 = call "Applied Send Command.vi"("error in (no error)"=w902, "Command"=T1."Feed to Length", "VISA resource name"=w903) -> ("error out"=w897:errorcluster, "VISA resource name out"=w901:refnum<visa-resource-name>)  [unwired: 4 in, 1 out]
            n503 = call "Time Delay15"("error in (no error)"=w897, "Delay Time (s)"=w899) -> ("error out"=w900:errorcluster)  [unwired: 9 in]
          }
        }
      }
      event "Jog X-": Mouse Up {
        n504 = event-data() -> ()  [unwired: 1 in, 8 out]
        n505 = flat-sequence {
          tunnel: [w918] -> w909
          tunnel: [w915] -> w907
          tunnel: [w914] -> w905
          tunnel: w913 -> [w920]
          tunnel: w912 -> [w919]
          tunnel: w909 -> [w929]
          tunnel: [w928] -> w908
          tunnel: w907 -> [w930]
          tunnel: [w931] -> w906
          tunnel: w905 -> [w927]
          tunnel: [w927] -> w904
          tunnel: w908 -> [w942]
          tunnel: w906 -> [w941]
          tunnel: [w940] -> w911
          tunnel: [w939] -> w910
          tunnel: w904 -> [w938]
          frame #0 {
            w914 = 0.1 ("Delay Time (s)")
            n506 = property on="X Velocity SP step/sec" class="DigNum (strict)"() -> ("Value"=w917:i32)  [unwired: 2 in, 2 out]
            n507 = property on="X steps/rev" class="DigNum (strict)"() -> ("Value"=w921:u32)  [unwired: 2 in, 2 out]
            n508 = Divide(x=w917, y=w921) -> (x/y=w922:dbl)
            n509 = Number To Fractional String(number=w922) -> (F-format string=w923:string)  [unwired: 3 in]
            n510 = call "Applied Send Command.vi"("error in (no error)"=w919, "Extra"=w923, "Command"=T1."Velocity Setting", "VISA resource name"=w920) -> ("error out"=w916:errorcluster, "VISA resource name out"=w918:refnum<visa-resource-name>)  [unwired: 3 in, 1 out]
            n511 = call "Time Delay6"("error in (no error)"=w916, "Delay Time (s)"=w914) -> ("error out"=w915:errorcluster)  [unwired: 9 in]
          }
          frame #1 {
            # "Distance/Position"
            n512 = property on="X Step SP" class="DigNum (strict)"() -> ("Value"=w932:i32)  [unwired: 2 in, 2 out]
            n513 = Multiply(x=-1, y=w932) -> (x*y=w926:i32)
            n514 = Number To Decimal String(number=w926) -> (decimal integer string=w934:string)  [unwired: 1 in]
            n515 = call "Applied Send Command.vi"("error in (no error)"=w930, "Extra"=w934, "Command"=T1."Distance or Position", "VISA resource name"=w929) -> ("error out"=w933:errorcluster, "VISA resource name out"=w928:refnum<visa-resource-name>)  [unwired: 3 in, 1 out]
            n516 = call "Time Delay7"("error in (no error)"=w933, "Delay Time (s)"=w927) -> ("error out"=w931:errorcluster)  [unwired: 9 in]
          }
          frame #2 {
            # "Feed to Position"
            n517 = call "Applied Send Command.vi"("error in (no error)"=w941, "Command"=T1."Feed to Length", "VISA resource name"=w942) -> ("error out"=w936:errorcluster, "VISA resource name out"=w940:refnum<visa-resource-name>)  [unwired: 4 in, 1 out]
            n518 = call "Time Delay5"("error in (no error)"=w936, "Delay Time (s)"=w938) -> ("error out"=w939:errorcluster)  [unwired: 9 in]
          }
        }
      }
      event Application Instance Close? {
        n519 = event-data() -> ()  [unwired: 1 in, 4 out]
        n520 = event-data() -> ()  [unwired: 3 in, 1 out]
      }
      event "Stop": Mouse Down {
        n521 = event-data() -> ()  [unwired: 1 in, 7 out]
        n522 = flat-sequence {
          tunnel: [w964] -> w952
          tunnel: [w963] -> w951
          tunnel: w950 -> [w965]
          tunnel: w949 -> [w962]
          frame #0 {
            n523 = call "Applied Send Command.vi"("error in (no error)"=w962, "Command"=T1."Stop", "VISA resource name"=w965) -> ("error out"=w963:errorcluster, "VISA resource name out"=w964:refnum<visa-resource-name>)  [unwired: 4 in, 1 out]
          }
        }
        n524 = flat-sequence {
          tunnel: w956 -> [w968]
          tunnel: w955 -> [w967]
          tunnel: [w969] -> w954
          tunnel: [w970] -> w953
          frame #0 {
            n525 = call "Applied Send Command.vi"("error in (no error)"=w967, "Command"=T1."Stop", "VISA resource name"=w968) -> ("error out"=w970:errorcluster, "VISA resource name out"=w969:refnum<visa-resource-name>)  [unwired: 4 in, 1 out]
          }
        }
        n526 = flat-sequence {
          tunnel: [w959] -> w946
          tunnel: [w960] -> w945
          tunnel: w948 -> [w957]
          tunnel: w947 -> [w958]
          frame #0 {
            n527 = call "Applied Send Command.vi"("error in (no error)"=w958, "Command"=T1."Stop", "VISA resource name"=w957) -> ("error out"=w960:errorcluster, "VISA resource name out"=w959:refnum<visa-resource-name>)  [unwired: 4 in, 1 out]
          }
        }
      }
      event "Reset": Mouse Down {
        n528 = event-data() -> ()  [unwired: 1 in, 7 out]
        n529 = flat-sequence {
          tunnel: [w991] -> w977
          tunnel: w978 -> [w993]
          tunnel: [w992] -> w976
          tunnel: w979 -> [w994]
          frame #0 {
            n530 = property on="Reset X Motor Steps" class="DigNum (strict)"() -> ("Value"=w997:i32)  [unwired: 2 in, 2 out]
            n531 = Number To Decimal String(number=w997) -> (decimal integer string=w995:string)  [unwired: 1 in]
            n532 = call "Applied Send Command.vi"("error in (no error)"=w993, "Extra"=w995, "Command"=T1."Set ABS Position", "VISA resource name"=w994) -> ("error out"=w992:errorcluster, "VISA resource name out"=w991:refnum<visa-resource-name>)  [unwired: 3 in, 1 out]
          }
        }
        n533 = flat-sequence {
          tunnel: w983 -> [w1002]
          tunnel: w982 -> [w999]
          tunnel: [w1001] -> w981
          tunnel: [w1000] -> w980
          frame #0 {
            n534 = property on="Reset Y Motor Steps" class="DigNum (strict)"() -> ("Value"=w1004:i32)  [unwired: 2 in, 2 out]
            n535 = Number To Decimal String(number=w1004) -> (decimal integer string=w1003:string)  [unwired: 1 in]
            n536 = call "Applied Send Command.vi"("error in (no error)"=w999, "Extra"=w1003, "Command"=T1."Set ABS Position", "VISA resource name"=w1002) -> ("error out"=w1000:errorcluster, "VISA resource name out"=w1001:refnum<visa-resource-name>)  [unwired: 3 in, 1 out]
          }
        }
        n537 = flat-sequence {
          tunnel: [w989] -> w973
          tunnel: [w988] -> w972
          tunnel: w975 -> [w986]
          tunnel: w974 -> [w987]
          frame #0 {
            n538 = property on="Reset Z Motor Steps" class="DigNum (strict)"() -> ("Value"=w990:i32)  [unwired: 2 in, 2 out]
            n539 = Number To Decimal String(number=w990) -> (decimal integer string=w984:string)  [unwired: 1 in]
            n540 = call "Applied Send Command.vi"("error in (no error)"=w987, "Extra"=w984, "Command"=T1."Set ABS Position", "VISA resource name"=w986) -> ("error out"=w988:errorcluster, "VISA resource name out"=w989:refnum<visa-resource-name>)  [unwired: 3 in, 1 out]
          }
        }
      }
    }
    n541 = local read "X Position mm PV"() -> (w268:dbl)
    n542 = local read "Y Position mm PV"() -> (w267:dbl)
    n543 = local read "Z Position mm PV"() -> (w269:dbl)
    n544 = Build Array("APX:PiezeX", "APX:PiezeY", "APX:PiezeZ") -> (w263:string[])
    n545 = Build Array(w268, w267, w269) -> (w262:dbl[])
    n546 = call-poly <userlib>:"CaLabPut.vi"("Values"=w262, "PV Names"=w263) -> ()  [unwired: 6 in, 4 out]
    n547 = case shown="True" "GFS" {
      tunnel: [0.0 ("data") 0.5 ("data")] -> w261
      frame False {
      }
      frame True {
      }
    }
    n548 = flat-sequence {
      tunnel: w261 -> [w296]
      frame #0 {
        w288 = 10 ("number of samples")
        n549 = call "DAQ Assistant2"("data"=w296) -> ()  [unwired: 17 in, 2 out]
        n550 = call "DAQ Assistant3"("number of samples"=w288) -> ("data"=w293:dynamicdata)  [unwired: 16 in, 2 out]
        n551 = call "Convert from Dynamic Data2"("Dynamic Data Type"=w293) -> ("Array"=w294:dbl[])  [unwired: 3 in]
        n552 = Add Array Elements(numeric array=w294) -> (sum=w292:dbl)
        n553 = Divide(x=w292, y=w288) -> (x/y=w291:dbl)
        n554 = Multiply(x=w296, y=0.8) -> (x*y=w289:dbl)
        n555 = Absolute Value(x=w291) -> (abs(x)=w295:dbl)
        "Dev5 Voltage 2" <- w295
        n556 = Greater?(x=w295, y=w289) -> (0:w297:bool)
        n557 = case shown="True" "Override 2" {
          tunnel: [w300 TRUE] -> w298
          tunnel: w297 -> [w300 _]
          frame False {
          }
          frame True {
          }
        }
        "NC" <- w298
      }
    }
  }
  n558 = flat-sequence {
    tunnel: w37 -> [w1006]
    tunnel: w36 -> [w1005]
    tunnel: [w1017] -> w21
    frame #0 {
      # "GET CURRENT POSITION"
      n559 = call "Applied Send Command.vi"("error in (no error)"=w1005, "Extra"="", "Command"=T1."Immediate Position?", "VISA resource name"=w1006) -> ("error out"=w1007:errorcluster, "read buffer"=w1012:string, "VISA resource name out"=w1008:refnum<visa-resource-name>)  [unwired: 3 in]
      n560 = call "Applied Send Command.vi"("error in (no error)"=w1007, "Command"=T1."Stop & Kill Buffer", "VISA resource name"=w1008) -> ("error out"=w1014:errorcluster, "VISA resource name out"=w1015:refnum<visa-resource-name>)  [unwired: 4 in, 1 out]
      n561 = Hexadecimal String To Number(string=w1012, offset=3) -> (number=w1009:u32)  [unwired: 1 in, 1 out]
      n562 = VISA Close(VISA resource name=w1015, error in (no error)=w1014) -> ()  [unwired: 1 out]
      n563 = To Long Integer(number=w1009) -> (32bit integer=w1017:i32)
    }
  }
  n564 = flat-sequence {
    tunnel: w23 -> [w1020]
    tunnel: w22 -> [w1019]
    tunnel: [w1018] -> w20
    frame #0 {
      # "GET CURRENT POSITION"
      n565 = call "Applied Send Command.vi"("error in (no error)"=w1019, "Extra"="", "Command"=T1."Immediate Position?", "VISA resource name"=w1020) -> ("error out"=w1021:errorcluster, "read buffer"=w1026:string, "VISA resource name out"=w1022:refnum<visa-resource-name>)  [unwired: 3 in]
      n566 = call "Applied Send Command.vi"("error in (no error)"=w1021, "Command"=T1."Stop & Kill Buffer", "VISA resource name"=w1022) -> ("error out"=w1028:errorcluster, "VISA resource name out"=w1029:refnum<visa-resource-name>)  [unwired: 4 in, 1 out]
      n567 = Hexadecimal String To Number(string=w1026, offset=3) -> (number=w1023:u32)  [unwired: 1 in, 1 out]
      n568 = VISA Close(VISA resource name=w1029, error in (no error)=w1028) -> ()  [unwired: 1 out]
      n569 = To Long Integer(number=w1023) -> (32bit integer=w1018:i32)
    }
  }
  n570 = flat-sequence {
    tunnel: w25 -> [w1032]
    tunnel: w24 -> [w1031]
    tunnel: [w1033] -> w19
    frame #0 {
      # "GET CURRENT POSITION"
      n571 = call "Applied Send Command.vi"("error in (no error)"=w1031, "Extra"="", "Command"=T1."Immediate Position?", "VISA resource name"=w1032) -> ("error out"=w1034:errorcluster, "read buffer"=w1039:string, "VISA resource name out"=w1035:refnum<visa-resource-name>)  [unwired: 3 in]
      n572 = call "Applied Send Command.vi"("error in (no error)"=w1034, "Command"=T1."Stop & Kill Buffer", "VISA resource name"=w1035) -> ("error out"=w1041:errorcluster, "VISA resource name out"=w1042:refnum<visa-resource-name>)  [unwired: 4 in, 1 out]
      n573 = Hexadecimal String To Number(string=w1039, offset=3) -> (number=w1036:u32)  [unwired: 1 in, 1 out]
      n574 = VISA Close(VISA resource name=w1042, error in (no error)=w1041) -> ()  [unwired: 1 out]
      n575 = To Long Integer(number=w1036) -> (32bit integer=w1033:i32)
    }
  }
  n576 = flat-sequence {
    tunnel: w21 -> [w1048]
    tunnel: w20 -> [w1047]
    tunnel: w19 -> [w1046]
    frame #0 {
      n577 = Build Array(w1048, w1047, w1046) -> (w1044:i32[])
      n578 = call-poly <vilib>:"Write To Spreadsheet File.vi"("1D data"=w1044, "file path (dialog if empty)"=path "S:/SSE/SCL2/POS.TXT") -> ()  [unwired: 6 in, 1 out]
    }
    frame #1 {
    }
  }
